vi "tui_LuaVIEW Task Manager.vi"() -> ()   [LabVIEW 2012]
doc: "This manager allows new tasks to be launched and existing tasks to be controlled and monitored. In case of a networked client/server setup, the tasks being managed are located on the server to which the client is connected."
uses:
  served/LuaVIEW Run or Swap Task_srv.ctl
  served/obj_LuaVIEW Task List_srv.ctl
  served/LuaVIEW Retrieve Scripts_srv.ctl
  served/LuaVIEW Info_srv.ctl
  served/re_LuaVIEW Kill Task_srv.ctl
  typedefs/t_LuaVIEW Task Manager Async Actions.ctl
  typedefs/t_LuaVIEW Task Manager States.ctl
  library/typedefs/t_Library Session Methods.ctl
  typedefs/clusters/LuaVIEW Task Console Ancillary.ctl
  typedefs/t_LuaVIEW Served Task List Methods.ctl
  typedefs/t_LuaVIEW Task Signals.ctl
  typedefs/t_LuaVIEW Task Modes.ctl
  clientsrv/typedefs/t_ClientSrv Access Levels.ctl
  library/glb_Library Configuration Globals.vi
panel:
  out "remote path cache":path
  out "remote file dialog":refnum<vi>
  in  "console":bool
  in  "swap remote":bool
  in  "swap local":bool
  in  "swap quick":bool
  out "kill task":T1
  in  "identifier":string
  out "info":T2
  out "retrieve scripts":T3
  in  "info":bool
  in  "run quick":bool
  in  "tabs":T4(tab)
  out "history content":string
  in  "insert new":bool
  in  "delete script":bool
  in  "next script":bool
  in  "previous script":bool
  in  "quick script history":string[](array[string])
  in  "script select":i32(ring)
  out "script":i32[](listbox)
  out "identifier":string
  in  "retrieve":bool
  out "handler":string
  out "swap time":string
  out "launch mode":enum16{"asynchronous", "manual", "synchronous"}(ring)
  out "deferred initialisation":bool
  out "priority":T5(ring)
  out "prefsys":T6(ring)
  out "task script on server":bool
  out "scripts":i32
  out "error":string
  in  "run remote":bool
  out "task list":T7
  out "run or swap task":T8
  out "local path cache":path
  in  "confirm":bool
  in  "kill":bool
  in  "run local":bool
  in  "stop":bool
  in  "resume":bool
  in  "pause":bool
  in  "task list":i32(listbox)
  in  "exit":bool
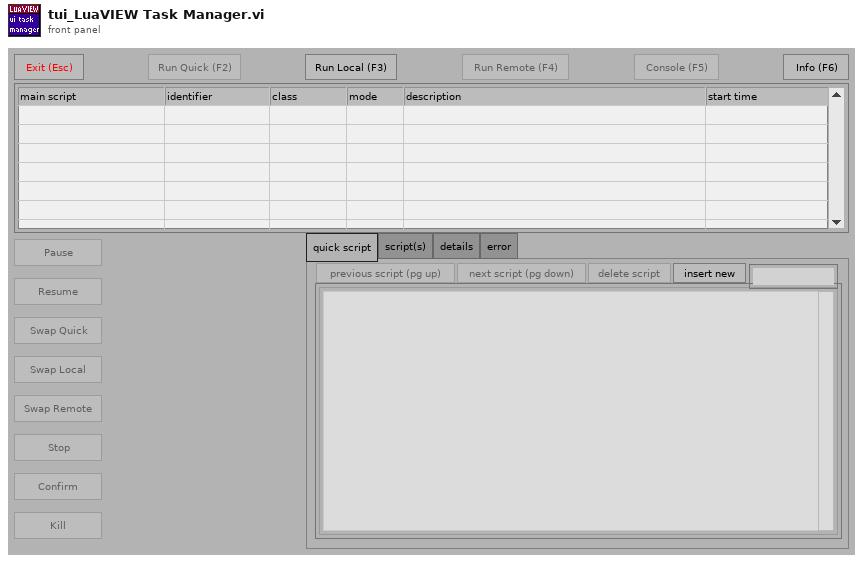
[diagram p1: front panel]
types:
  T1 = typedef "re_LuaVIEW Kill Task_srv.ctl" = refnum<vi>
  T2 = typedef "LuaVIEW Info_srv.ctl" = refnum<vi>
  T3 = typedef "LuaVIEW Retrieve Scripts_srv.ctl" = refnum<vi>
  T4 = enum32{"quick script", "script(s)", "details", "error"}
  T5 = enum32{"invalid priority", "background priority", "normal priority", "above normal priority", "high priority", "time critical priority", "subroutine"}
  T6 = enum32{"invalid execution system", "user interface", "standard", "instrument i/o", "data acquisition", "other 1", "other 2", "same as caller"}
  T7 = typedef "obj_LuaVIEW Task List_srv.ctl" = refnum<vi>
  T8 = typedef "LuaVIEW Run or Swap Task_srv.ctl" = refnum<vi>
  T9 = typedef "t_LuaVIEW Task Manager States.ctl" = enum16{"empty queue", "poll list", "reselect", "select", "resize", "pause task", "resume task", "stop task", "confirm error", "swap quick", "swap local", "swap remote", "kill task", "retrieve scripts", "select script", "quick ablement", "initialize", "init refs", "init remote dlg", "init persist", "init list", "init scripts", "cleanup", "stop"}
  T10 = typedef "t_LuaVIEW Task Manager Async Actions.ctl" = enum16{"run quick", "run local", "run remote", "stop"}
  T11 = typedef "t_ClientSrv Access Levels.ctl" = enum16{"observer", "operator", "local"}
  T12 = enum32{"existing file", "new file", "new or existing file", "existing dir", "new dir", "new or existing dir", "existing file (use LLBs)", "new file (use LLBs)", "new or existing file (use LLBs)", "new or existing file or directory (use LLBs)"}
  T13 = typedef "t_Library Session Methods.ctl" = enum16{"run", "get arg", "set arg", "delist", "cleanup?", "start session", "stop session", "list empty?"}
  T14 = typedef "LuaVIEW Task Console Ancillary.ctl" = cluster{"open on start":bool, "stop on close":bool, "hide initial":bool, "timeout":u32}
  T15 = typedef "t_LuaVIEW Served Task List Methods.ctl" = enum16{"get list", "resume", "pause", "swap", "stop", "confirm"}
  T16 = typedef "t_LuaVIEW Task Signals.ctl" = enum32{"resume", "pause", "swap", "stop", "confirm"}
  T17 = typedef "t_LuaVIEW Task Modes.ctl" = enum16{"initializing", "running", "executing", "paused", "error", "swapping"}
  T18 = typedef "eventvkey.ctl" = enum16{"ASCII", "Enter", "Return", "Shift", "Ctrl", "Alt", "Cmd", "Opt", "Caps", "NumLock", "Clear", "Break", "Up", "Down", "Left", "Right", "Insert", "Delete", "Home", "End", "PageUp", "PageDown", "Escape", "Help", "Pause", "ScrollLock", "F1", "F2", "F3", "F4", "F5", "F6", "F7", "F8", "F9", "F10", "F11", "F12", "F13", "F14", "F15", "F16", "F17", "F18", "F19", "F20", "F21", "F22", "F23", "F24", "Play", "VolumeUp", "VolumeDown", "Mute", "Two Byte Char"}
  T19 = typedef "LuaVIEW Task Info.ctl" = cluster{"main script":string, "identifier":string, "class":string, "description":string, "mode":T17, "handler":string, "LuaVIEW reference":T20, "scripts":i32, "hide":bool, "active":bool, "error msg":string, "defer":bool, "launch":enum16{"asynchronous", "manual", "synchronous"}, "main path valid":bool, "start time":dbl, "swap time":dbl, "task VI":refnum<vi>, "prefsys":enum32{"invalid execution system", "user interface", "standard", "instrument i/o", "data acquisition", "other 1", "other 2", "same as caller"}, "priority":enum32{"invalid priority", "background priority", "normal priority", "above normal priority", "high priority", "time critical priority", "subroutine"}, "signal flags":u32, "allow mask":u32, "handle mask":u32, "disallow manual":bool}
  T20 = typedef "t_LuaVIEW Reference.ctl" = refnum<k1>
  T21 = typedef "LuaVIEW Script Info.ctl" = cluster{"path":path, "description":string, "text":string, "parent index":i32, "version":string}
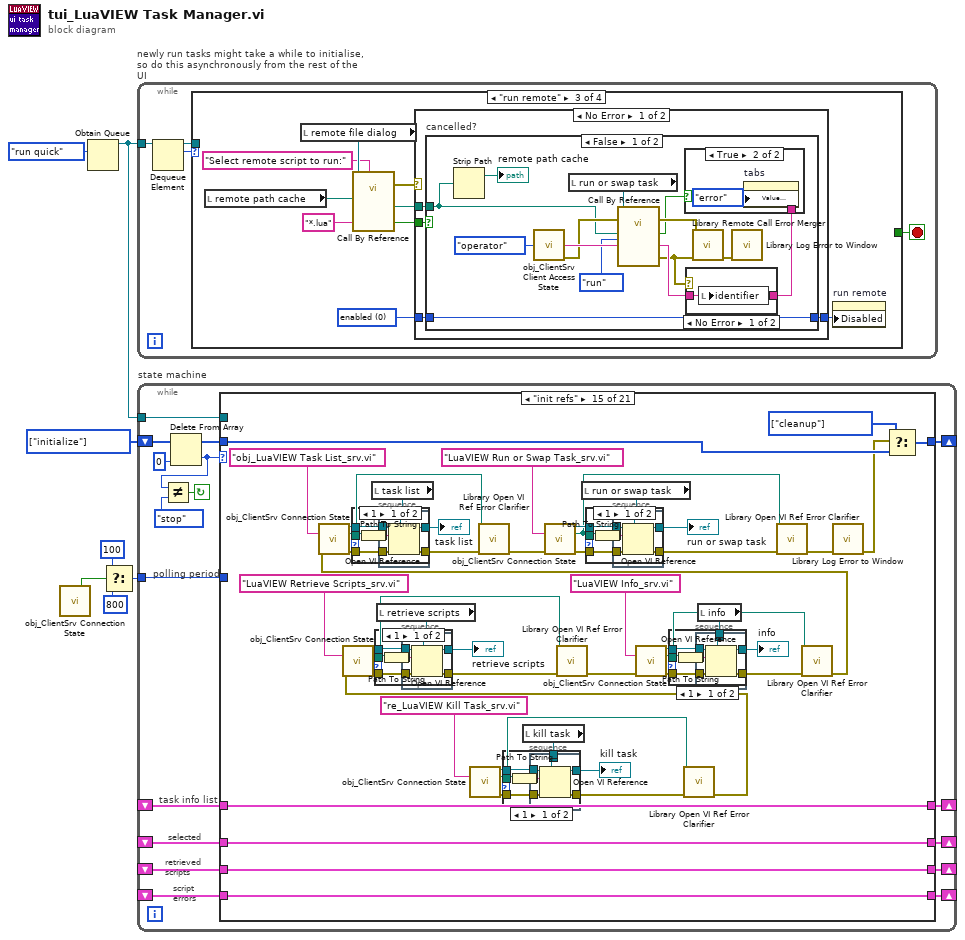
[diagram p0: block diagram]
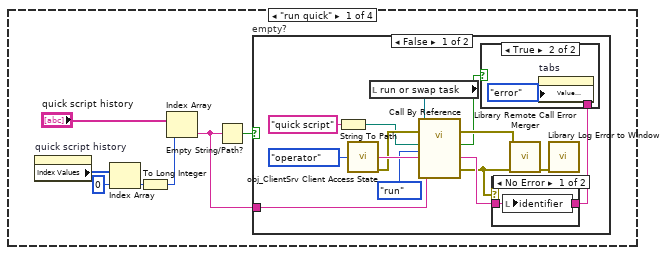
[diagram p2: hidden frame]
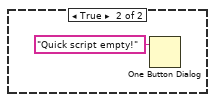
[diagram p5: hidden frame]
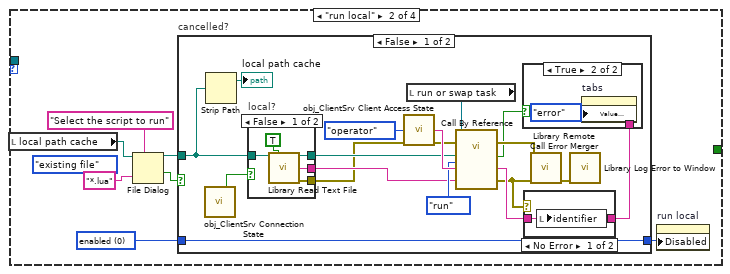
[diagram p6: hidden frame]
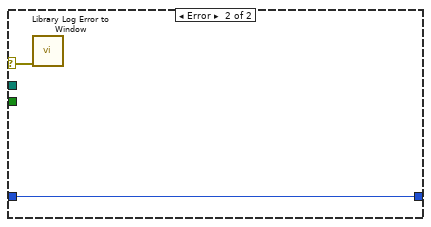
[diagram p14: hidden frame]
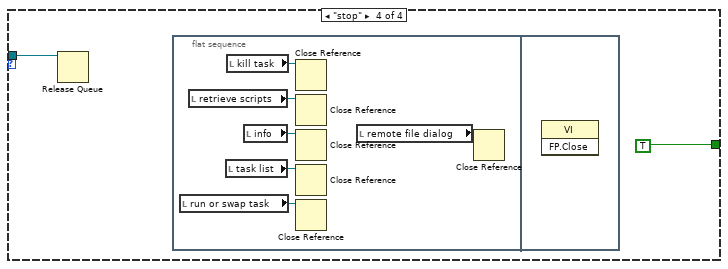
[diagram p15: hidden frame]
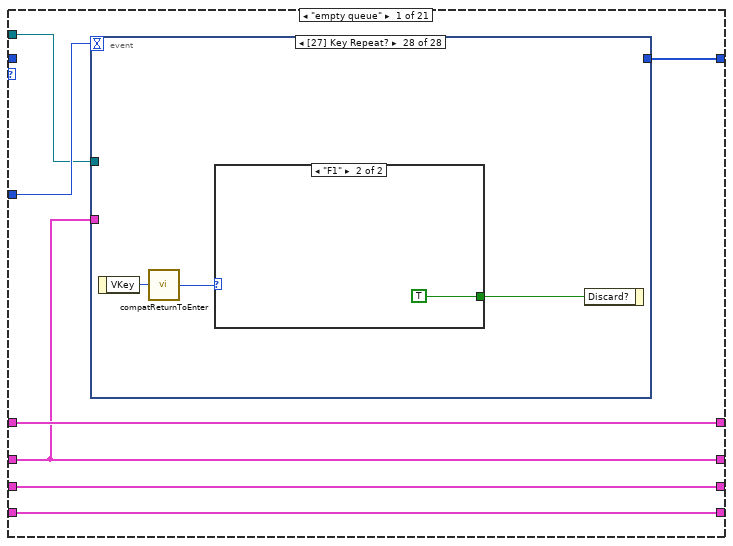
[diagram p16: hidden frame]
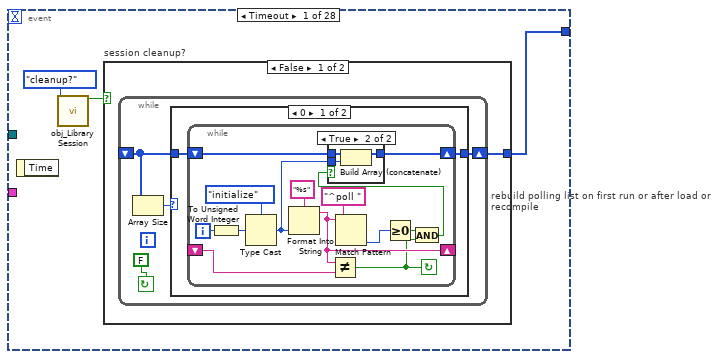
[diagram p17: hidden frame]
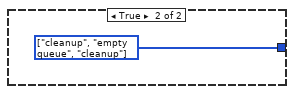
[diagram p20: hidden frame]
diagram:
  w7 = T9[] [enum."initialize"] items=["empty queue", "poll list", "reselect", "select", "resize", "pause task", "resume task", "stop task", "confirm error", "swap quick", "swap local", "swap remote", "kill task", "retrieve scripts", "select script", "quick ablement", "initialize", "init refs", "init remote dlg", "init persist", "init list", "init scripts", "cleanup", "stop"] ("Array Constant")
  n1 = call "obj_ClientSrv Connection State.vi"() -> ("local?"=w3:bool)  [unwired: 8 in, 7 out]
  n2 = Obtain Queue(element data type=t_LuaVIEW_Task_Manager_Async_Actions."run quick" ("actions")) -> (queue out=w6:refnum<queue>)  [unwired: 4 in, 2 out]
  n3 = Select(t=100, s=w3, f=800) -> (s? t:f=w2:i32)
  n4 = while "newly run tasks might take a while to initialise, so do this asynchronously from the rest of the UI" {
    tunnel: w6 -> [w11]
    stop <- w9 stop-if-true
    n5 = Dequeue Element(queue=w11) -> (queue out=w10:refnum<queue>, element=w8:T10)  [unwired: 2 in, 2 out]
    n6 = case "Case" shown="\"run remote\"" w8 {
      tunnel: w10 -> [_ _ _ w106]
      tunnel: [_ _ _ TRUE] -> w9
      frame "run quick" {
        n7 = property on="quick script history" class="Arr (strict)"() -> ("Index Values"=w18:u32[])  [unwired: 2 in, 2 out]
        n8 = Index Array(array=w18, index=0) -> (element=w15:u32)
        n9 = To Long Integer(number=w15) -> (32bit integer=w14:i32)
        n10 = Index Array(array="quick script history", index=w14) -> (element=w12:string)
        n11 = Empty String/Path?(string/path=w12) -> (empty?=w13:bool)
        n12 = case "empty?" shown="False" w13 {
          tunnel: w12 -> [w26 _]
          frame False {
            n13 = String To Path(string="quick script") -> (path=w24:path)
            n14 = call "obj_ClientSrv Client Access State.vi"("access level (observer)"=t_ClientSrv_Access_Levels."operator" ("access level in")) -> ("certificate"=w29:string, "error out"=w28:errorcluster)  [unwired: 13 in]
            n15 = local read "run or swap task"() -> (w27:T8)
            n16 = call-by-ref "?"(reference=w27, error in=w28, "script file or name (no name)"=w24, "action"=enum16{"run", "swap"}."run", "certificate"=w29, "script string (\"\" == load from file)"=w26) -> (error out=w32:errorcluster, "manual error"=w22:bool, "identifier"=w23:string, 15:"error out"=w21:errorcluster)  [unwired: 9 in, 1 out]
            n17 = case shown="No Error" w21 {
              tunnel: w23 -> [w33 w34]
              tunnel: [w33 w34] -> w20
              frame No Error {
                n18 = local write "identifier"(w33) -> ()
              }
              frame Error {
              }
            }
            n19 = case shown="True" w22 {
              tunnel: w20 -> [_ _]
              frame False {
              }
              frame True {
                n20 = property on="tabs" class="TabCtl (strict)"("Value (Signaling)"=T4."error") -> ()  [unwired: 2 in, 2 out]
              }
            }
            n21 = call "Library Remote Call Error Merger.vi"("call by reference node error"=w32, "called VI error (no error)"=w21) -> ("error out"=w31:errorcluster)  [unwired: 13 in]
            n22 = call "Library Log Error to Window.vi"("error in (no error)"=w31) -> ()  [unwired: 13 in, 2 out]
          }
          frame True {
            n23 = One Button Dialog(message="Quick script empty!") -> ()  [unwired: 1 in, 1 out]
          }
        }
      }
      frame "run local" {
        w37 = u8 0 items=["enabled", "disabled", "grayed"] ("disabled state")
        (unwired) T12."existing file" ("select mode (2)")
        n24 = local read "local path cache"() -> (w39:path)
        n25 = File Dialog(6:"*.lua" ("pattern"), 7:"Select the script to run" ("prompt (default)"), 11:w39) -> (1:w40:bool, 3:w41:path)  [unwired: 4 in, 2 out]
        n26 = case "cancelled?" shown="False" w40 {
          tunnel: w41 -> [w48 _]
          tunnel: w37 -> [w60 w71]
          tunnel: [w60 w71] -> w38
          frame False {
            n27 = call "obj_ClientSrv Connection State.vi"() -> ("local?"=w44:bool)  [unwired: 8 in, 7 out]
            n28 = Strip Path(path=w48) -> (stripped path=→"local path cache":path)  [unwired: 1 out]
            n29 = case "local?" shown="False" w44 {
              tunnel: w48 -> [w66 w67]
              tunnel: [w64 w67] -> w47
              tunnel: [w63 _] -> w46
              tunnel: [w62 _] -> w45
              frame False {
                n30 = call "Library Read Text File.vi"("file path"=w66, "convert eol (F)"=TRUE) -> ("dup path"=w64:path, "read text"=w63:string, "error out"=w62:errorcluster)  [unwired: 11 in]
              }
              frame True {
              }
            }
            n31 = call "obj_ClientSrv Client Access State.vi"("access level (observer)"=t_ClientSrv_Access_Levels."operator" ("access level in"), "error in (no error)"=w45) -> ("certificate"=w56:string, "error out"=w55:errorcluster)  [unwired: 12 in]
            n32 = local read "run or swap task"() -> (w54:T8)
            n33 = call-by-ref "?"(reference=w54, error in=w55, "script file or name (no name)"=w47, "action"=enum16{"run", "swap"}."run", "certificate"=w56, "script string (\"\" == load from file)"=w46) -> (error out=w59:errorcluster, "manual error"=w52:bool, "identifier"=w53:string, 15:"error out"=w50:errorcluster)  [unwired: 9 in, 1 out]
            n34 = case shown="No Error" w50 {
              tunnel: w53 -> [w68 w69]
              tunnel: [w68 w69] -> w51
              frame No Error {
                n35 = local write "identifier"(w68) -> ()
              }
              frame Error {
              }
            }
            n36 = case shown="True" w52 {
              tunnel: w51 -> [_ _]
              frame False {
              }
              frame True {
                n37 = property on="tabs" class="TabCtl (strict)"("Value (Signaling)"=T4."error") -> ()  [unwired: 2 in, 2 out]
              }
            }
            n38 = call "Library Remote Call Error Merger.vi"("call by reference node error"=w59, "called VI error (no error)"=w50) -> ("error out"=w58:errorcluster)  [unwired: 13 in]
            n39 = call "Library Log Error to Window.vi"("error in (no error)"=w58) -> ()  [unwired: 13 in, 2 out]
          }
          frame True {
          }
        }
        n40 = property on="run local" class="Bool"("Disabled"=w38) -> ()  [unwired: 2 in, 2 out]
      }
      frame "run remote" {
        w79 = u8 0 items=["enabled", "disabled", "grayed"] ("disabled state")
        n41 = local read "remote path cache"() -> (w75:path)
        n42 = local read "remote file dialog"() -> (w78:refnum<vi>)
        n43 = call-by-ref "?"(reference=w78, "prompt"="Select remote script to run:" ("prompt (default)"), "pattern"="*.lua", "start path"=w75) -> (error out=w77:errorcluster, "cancelled"=w74:bool, "path"=w72:path)  [unwired: 8 in, 1 out]
        n44 = case shown="No Error" w77 {
          selector: w77 -> [_ w103]
          tunnel: [w84 w104] -> w80
          tunnel: w79 -> [w83 w104]
          tunnel: w74 -> [w82 _]
          tunnel: w72 -> [w81 _]
          frame No Error {
            n45 = case "cancelled?" shown="False" w82 {
              tunnel: w83 -> [w97 w102]
              tunnel: [w97 w102] -> w84
              tunnel: w81 -> [w85 _]
              frame False {
                n46 = Strip Path(path=w85) -> (stripped path=→"remote path cache":path)  [unwired: 1 out]
                n47 = call "obj_ClientSrv Client Access State.vi"("access level (observer)"=t_ClientSrv_Access_Levels."operator" ("access level in")) -> ("certificate"=w93:string, "error out"=w92:errorcluster)  [unwired: 13 in]
                n48 = local read "run or swap task"() -> (w91:T8)
                n49 = call-by-ref "?"(reference=w91, error in=w92, "script file or name (no name)"=w85, "action"=enum16{"run", "swap"}."run", "certificate"=w93) -> (error out=w96:errorcluster, "manual error"=w89:bool, "identifier"=w90:string, 15:"error out"=w87:errorcluster)  [unwired: 10 in, 1 out]
                n50 = case shown="No Error" w87 {
                  tunnel: w90 -> [w99 w100]
                  tunnel: [w99 w100] -> w88
                  frame No Error {
                    n51 = local write "identifier"(w99) -> ()
                  }
                  frame Error {
                  }
                }
                n52 = case shown="True" w89 {
                  tunnel: w88 -> [_ _]
                  frame False {
                  }
                  frame True {
                    n53 = property on="tabs" class="TabCtl (strict)"("Value (Signaling)"=T4."error") -> ()  [unwired: 2 in, 2 out]
                  }
                }
                n54 = call "Library Remote Call Error Merger.vi"("call by reference node error"=w96, "called VI error (no error)"=w87) -> ("error out"=w95:errorcluster)  [unwired: 13 in]
                n55 = call "Library Log Error to Window.vi"("error in (no error)"=w95) -> ()  [unwired: 13 in, 2 out]
              }
              frame True {
              }
            }
          }
          frame Error {
            n56 = call "Library Log Error to Window.vi"("error in (no error)"=w103) -> ()  [unwired: 13 in, 2 out]
          }
        }
        n57 = property on="run remote" class="Bool"("Disabled"=w80) -> ()  [unwired: 2 in, 2 out]
      }
      frame "stop" {
        n58 = Release Queue(queue=w106) -> ()  [unwired: 2 in, 3 out]
        n59 = flat-sequence {
          frame #0 {
            n60 = local read "run or swap task"() -> (w111:T8)
            n61 = local read "retrieve scripts"() -> (w110:T3)
            n62 = local read "task list"() -> (w112:T7)
            n63 = local read "kill task"() -> (w108:T1)
            n64 = local read "info"() -> (w109:T2)
            n65 = Close Reference(reference=w108) -> ()  [unwired: 1 in, 1 out]
            n66 = Close Reference(reference=w110) -> ()  [unwired: 1 in, 1 out]
            n67 = Close Reference(reference=w109) -> ()  [unwired: 1 in, 1 out]
            n68 = Close Reference(reference=w112) -> ()  [unwired: 1 in, 1 out]
            n69 = Close Reference(reference=w111) -> ()  [unwired: 1 in, 1 out]
            n70 = local read "remote file dialog"() -> (w107:refnum<vi>)
            n71 = Close Reference(reference=w107) -> ()  [unwired: 1 in, 1 out]
          }
          frame #1 {
            n72 = invoke class="VI" method="FP.Close"() -> ()  [unwired: 3 in, 3 out]
          }
        }
      }
    }
  }
  n73 = while "state machine" {
    shift-left: w7 -> [w126]
    shift-right: [w129] -> _
    shift-right: [w122] -> _
    shift-left: _ -> [w123]
    shift-right: [w120] -> _
    shift-left: _ -> [w121]
    tunnel: w6 -> [w119]
    tunnel: w2 -> [w118]
    shift-right: [w116] -> _
    shift-left: _ -> [w117]
    shift-right: [w115] -> _
    shift-left: _ -> [w114]
    stop <- w128 continue-if-true
    # "script\nerrors"
    # "retrieved\nscripts"
    # "polling period"
    # "selected"
    # "task info list"
    n74 = Delete From Array(array=w126, index=0) -> (deleted portion=w113:T9, array with subset deleted=w125:T9[])  [unwired: 1 in]
    n75 = Not Equal?(x=w113, y=t_LuaVIEW_Task_Manager_States."stop" ("states")) -> (x != y?=w128:bool)
    n76 = case "Case" shown="\"init refs\"" w113 {
      selector: w113 -> [_ _ _ _ _ w563 _ _ _ _ _ _ _ _ _ _ _ _ _ _ _]
      tunnel: [w136 w351 w424 w438 w558 w574 w590 w622 w656 w676 w696 w734 w759 w780 w855 w962 w981 w989 w1002 w1018 w1027] -> w129
      tunnel: w125 -> [_ w352 w425 w438 w558 w574 w590 w622 w656 w677 w708 w734 w759 _ w853 w962 w982 w990 w1003 _ w1027]
      tunnel: w123 -> [w135 w358 w420 w437 w560 w575 w589 w621 w655 w678 w709 w733 w761 w782 w852 w968 w985 w992 w1005 w1012 w1026]
      tunnel: [w135 w359 w420 w437 w560 w575 w589 w621 w655 w678 w709 w733 w761 w782 w852 w968 w985 w992 w1005 w1012 w1020] -> w122
      tunnel: w121 -> [w130 w357 w426 _ w559 w561 w586 w613 w652 w675 w694 w732 w760 w781 w851 w967 w984 w991 w1004 w1017 w1025]
      tunnel: [w130 w357 w426 w435 w559 w561 w586 w613 w652 w675 w694 w732 w760 w781 w851 w967 w984 w991 w1004 w1017 w1025] -> w120
      tunnel: w119 -> [w131 _ _ _ _ _ _ _ _ _ _ _ _ _ _ _ _ _ _ _ w1024]
      tunnel: w118 -> [w134 _ _ _ _ _ _ _ _ _ _ _ _ _ _ _ _ _ _ _ _]
      tunnel: w117 -> [w133 w346 w422 w434 w556 w566 w588 w620 w654 w680 _ w731 w741 w779 w847 w966 w979 w987 w1000 w1014 w1023]
      tunnel: [w133 w346 w422 w434 w556 w566 w588 w620 w654 w680 w700 w731 w741 w779 w847 w966 w979 w987 w996 w1014 w1023] -> w116
      tunnel: [w132 w345 w421 w433 w555 w565 w587 w619 w653 w679 w699 w729 w740 w778 w845 w965 w978 w986 w994 w1013 w1022] -> w115
      tunnel: w114 -> [w132 w345 w421 w433 w555 w565 w587 w619 w653 w679 _ w729 w740 w778 w845 w965 w978 w986 w999 w1013 w1022]
      frame "empty queue" {
        n77 = event shown="[27] Key Repeat?" {
          selector: _ -> [_ _ _ _ _ _ _ _ _ _ _ _ _ _ _ _ _ _ _ _ _ _ _ _ _ _ _ _]
          dyn-events: _ -> [_ _ _ _ _ _ _ _ _ _ _ _ _ _ _ _ _ _ _ _ _ _ _ _ _ _ _ _]
          timeout: w134 -> [_ _ _ _ _ _ _ _ _ _ _ _ _ _ _ _ _ _ _ _ _ _ _ _ _ _ _ _]
          tunnel: [w139 w168 w170 _ w176 w179 w183 _ _ _ _ w222 w229 w236 w243 w251 w253 w266 w276 w292 w312 w314 w322 w323 w324 w325 w328 _] -> w136
          tunnel: w131 -> [_ _ _ w172 _ _ _ w185 w194 _ _ _ _ _ _ _ _ _ _ _ _ _ _ _ _ _ _ _]
          tunnel: w130 -> [_ _ _ _ _ _ _ _ _ w201 _ _ _ _ _ _ _ _ _ _ _ _ _ _ _ _ _ _]
          event Timeout {
            n78 = event-data() -> ()  [unwired: 1 in, 1 out]
            n79 = call "obj_Library Session.vi"("method"=t_Library_Session_Methods."cleanup?") -> ("cleanup/empty?"=w138:bool)  [unwired: 11 in, 3 out]
            n80 = case "session cleanup?" shown="False" w138 {
              tunnel: [w140 w166] -> w139
              frame False {
                n81 = while "rebuild polling list on first run or after load or recompile" {
                  shift-left: _ -> [w143]
                  shift-right: [w142] -> w140
                  stop <- FALSE continue-if-true
                  n82 = Array Size(array=w143) -> (size(s)=w144:i32)
                  n83 = case shown="0" w144 {
                    tunnel: [w145 w165] -> w142
                    tunnel: w143 -> [w146 w165]
                    frame 0 {
                      n84 = while {
                        shift-left: w146 -> [w155]
                        shift-right: [w153] -> w145
                        shift-left: _ -> [w157]
                        shift-right: [w152] -> _
                        i -> [w160]
                        stop <- w148 continue-if-true
                        n85 = To Unsigned Word Integer(number=w160) -> (unsigned 16bit integer=w158:u16)
                        n86 = Type Cast(type=t_LuaVIEW_Task_Manager_States."initialize" ("states"), x=w158) -> (*(type *) &x=w154:T9)
                        n87 = Format Into String(format string="%s" ("Format String"), w154) -> (resulting string=w152:string)  [unwired: 2 in, 1 out]
                        n88 = Not Equal?(x=w152, y=w157) -> (x != y?=w148:bool)
                        n89 = Match Pattern(string=w152, regular expression="^poll ") -> (offset past match=w150:i32)  [unwired: 1 in, 3 out]
                        n90 = Greater Or Equal To 0?(x=w150) -> (x >= 0?=w149:bool)
                        n91 = And(x=w149, y=w148) -> (x .and. y?=w147:bool)
                        n92 = case shown="True" w147 {
                          tunnel: w155 -> [w161 w164]
                          tunnel: w154 -> [_ w163]
                          tunnel: [w161 w162] -> w153
                          frame False {
                          }
                          frame True {
                            n93 = Build Array (concatenate)(w164, w163) -> (w162:T9[])
                          }
                        }
                      }
                    }
                    frame Default {
                    }
                  }
                }
              }
              frame True {
                w166 = T9[] [enum."cleanup", enum."empty queue", enum."cleanup"] items=["empty queue", "poll list", "reselect", "select", "resize", "pause task", "resume task", "stop task", "confirm error", "swap quick", "swap local", "swap remote", "kill task", "retrieve scripts", "select script", "quick ablement", "initialize", "init refs", "init remote dlg", "init persist", "init list", "init scripts", "cleanup", "stop"] ("Array Constant")
              }
            }
          }
          event Panel Close? {
            w168 = T9[] [enum."cleanup"] items=["empty queue", "poll list", "reselect", "select", "resize", "pause task", "resume task", "stop task", "confirm error", "swap quick", "swap local", "swap remote", "kill task", "retrieve scripts", "select script", "quick ablement", "initialize", "init refs", "init remote dlg", "init persist", "init list", "init scripts", "cleanup", "stop"] ("Array Constant")
            n94 = event-data() -> ()  [unwired: 1 in, 3 out]
            n95 = event-data("Discard?"=TRUE) -> ()  [unwired: 1 in, 1 out]
          }
          event "exit": Value Change {
            n96 = event-data() -> ()  [unwired: 1 in, 1 out]
            n97 = case shown="True" "exit" {
              tunnel: [w171 _] -> w170
              frame True {
                w171 = T9[] [enum."cleanup", enum."empty queue", enum."cleanup"] items=["empty queue", "poll list", "reselect", "select", "resize", "pause task", "resume task", "stop task", "confirm error", "swap quick", "swap local", "swap remote", "kill task", "retrieve scripts", "select script", "quick ablement", "initialize", "init refs", "init remote dlg", "init persist", "init list", "init scripts", "cleanup", "stop"] ("Array Constant")
              }
              frame False {
              }
            }
          }
          event "run quick": Value Change {
            n98 = event-data() -> ()  [unwired: 1 in, 5 out]
            n99 = case shown="True" "run quick" {
              tunnel: w172 -> [w175 _]
              frame True {
                n100 = Enqueue Element(queue=w175, element=t_LuaVIEW_Task_Manager_Async_Actions."run quick" ("states")) -> ()  [unwired: 2 in, 3 out]
              }
              frame False {
              }
            }
          }
          event "swap quick": Value Change {
            n101 = event-data() -> ()  [unwired: 1 in, 1 out]
            n102 = case shown="True" "swap quick" {
              tunnel: [w178 _] -> w176
              frame True {
                w178 = T9[] [enum."swap quick"] items=["empty queue", "poll list", "reselect", "select", "resize", "pause task", "resume task", "stop task", "confirm error", "swap quick", "swap local", "swap remote", "kill task", "retrieve scripts", "select script", "quick ablement", "initialize", "init refs", "init remote dlg", "init persist", "init list", "init scripts", "cleanup", "stop"] ("Array Constant")
              }
              frame False {
              }
            }
          }
          event "swap local": Value Change {
            n103 = event-data() -> ()  [unwired: 1 in, 1 out]
            n104 = case shown="True" "swap local" {
              tunnel: [w181 _] -> w179
              frame True {
                w181 = T9[] [enum."swap local"] items=["empty queue", "poll list", "reselect", "select", "resize", "pause task", "resume task", "stop task", "confirm error", "swap quick", "swap local", "swap remote", "kill task", "retrieve scripts", "select script", "quick ablement", "initialize", "init refs", "init remote dlg", "init persist", "init list", "init scripts", "cleanup", "stop"] ("Array Constant")
              }
              frame False {
              }
            }
          }
          event "swap remote": Value Change {
            n105 = event-data() -> ()  [unwired: 1 in, 1 out]
            n106 = case shown="True" "swap remote" {
              tunnel: [w184 _] -> w183
              frame True {
                w184 = T9[] [enum."swap remote"] items=["empty queue", "poll list", "reselect", "select", "resize", "pause task", "resume task", "stop task", "confirm error", "swap quick", "swap local", "swap remote", "kill task", "retrieve scripts", "select script", "quick ablement", "initialize", "init refs", "init remote dlg", "init persist", "init list", "init scripts", "cleanup", "stop"] ("Array Constant")
              }
              frame False {
              }
            }
          }
          event "run local": Value Change {
            n107 = event-data() -> ()  [unwired: 1 in, 5 out]
            n108 = case shown="True" "run local" {
              tunnel: w185 -> [w188 _]
              frame True {
                n109 = flat-sequence {
                  tunnel: w188 -> [w190]
                  tunnel: [w190] -> w187
                  tunnel: w187 -> [w192]
                  frame #0 {
                    w189 = u8 2 items=["enabled", "disabled", "grayed"] ("disabled state")
                    n110 = property on="run local" class="Bool"("Disabled"=w189) -> ()  [unwired: 2 in, 2 out]
                  }
                  frame #1 {
                    n111 = Enqueue Element(queue=w192, element=t_LuaVIEW_Task_Manager_Async_Actions."run local" ("states")) -> ()  [unwired: 2 in, 3 out]
                  }
                }
              }
              frame False {
              }
            }
          }
          event "run remote": Value Change {
            n112 = event-data() -> ()  [unwired: 1 in, 1 out]
            n113 = case shown="True" "run remote" {
              tunnel: w194 -> [w196 _]
              frame True {
                n114 = flat-sequence {
                  tunnel: w196 -> [w198]
                  tunnel: [w198] -> w195
                  tunnel: w195 -> [w200]
                  frame #0 {
                    w197 = u8 2 items=["enabled", "disabled", "grayed"] ("disabled state")
                    n115 = property on="run remote" class="Bool"("Disabled"=w197) -> ()  [unwired: 2 in, 2 out]
                  }
                  frame #1 {
                    n116 = Enqueue Element(queue=w200, element=t_LuaVIEW_Task_Manager_Async_Actions."run remote" ("states")) -> ()  [unwired: 2 in, 3 out]
                  }
                }
              }
              frame False {
              }
            }
          }
          event "console": Value Change {
            n117 = event-data() -> ()  [unwired: 1 in, 5 out]
            n118 = case shown="True" "console" {
              tunnel: w201 -> [w206 _]
              frame True {
                n119 = Unbundle By Name(w206) -> ("identifier"=w205:string)
                n120 = call "Library Resolve VI Path.vi"("VI name"="ui_LuaVIEW Task Console.vit", "sub path of toolkit (none)"=path "dynamic" ("subdirectory of tree (none)")) -> ("VI path"=w207:path)  [unwired: 13 in]
                n121 = Flatten To String(anything=T14 {"open on start"=TRUE, "stop on close"=TRUE, "hide initial"=FALSE, "timeout"=0} ("task console ancillary")) -> (data string=w203:string)  [unwired: 3 in, 2 out]
                n122 = call "obj_Library Session.vi"("method"=t_Library_Session_Methods."run", "path"=w207, "argument in (none)"=w205, "ancillary in (none)"=w203) -> ("error out"=w208:errorcluster)  [unwired: 8 in, 3 out]
                n123 = call "Library Log Error to Window.vi"("error in (no error)"=w208) -> ()  [unwired: 13 in, 2 out]
              }
              frame False {
              }
            }
          }
          event "info": Value Change {
            n124 = event-data() -> ()  [unwired: 1 in, 5 out]
            n125 = case shown="True" "info" {
              frame True {
                n126 = call "obj_ClientSrv Client Access State.vi"() -> ("certificate"=w218:string, "error out"=w217:errorcluster)  [unwired: 14 in]
                n127 = local read "info"() -> (w219:T2)
                n128 = call-by-ref "?"(reference=w219, error in=w217, "certificate"=w218) -> (error out=w215:errorcluster, "info"=w213:string, 15:"error out"=w216:errorcluster)  [unwired: 13 in, 1 out]
                n129 = call "Library Remote Call Error Merger.vi"("call by reference node error"=w215, "called VI error (no error)"=w216) -> ("error out"=w214:errorcluster)  [unwired: 13 in]
                n130 = case shown="No Error" w214 {
                  selector: w214 -> [_ w221]
                  tunnel: w213 -> [w220 _]
                  frame No Error {
                    n131 = One Button Dialog(message=w220) -> ()  [unwired: 1 in, 1 out]
                  }
                  frame Error {
                    n132 = call "Library Log Error to Window.vi"("error in (no error)"=w221) -> ()  [unwired: 13 in, 2 out]
                  }
                }
              }
              frame False {
              }
            }
          }
          event "pause": Value Change {
            n133 = event-data() -> ()  [unwired: 1 in, 5 out]
            n134 = case shown="True" "pause" {
              tunnel: [w227 _] -> w222
              frame True {
                w226 = u8 0 items=["enabled", "disabled", "grayed"] ("disabled state")
                n135 = property on="pause" class="Bool"() -> ("Disabled"=w225:u8)  [unwired: 2 in, 2 out]
                n136 = Equal?(x=w225, y=w226) -> (x = y?=w224:bool)
                n137 = case shown="True" w224 {
                  tunnel: [_ w228] -> w227
                  frame False {
                  }
                  frame True {
                    w228 = T9[] [enum."pause task"] items=["empty queue", "poll list", "reselect", "select", "resize", "pause task", "resume task", "stop task", "confirm error", "swap quick", "swap local", "swap remote", "kill task", "retrieve scripts", "select script", "quick ablement", "initialize", "init refs", "init remote dlg", "init persist", "init list", "init scripts", "cleanup", "stop"] ("Array Constant")
                  }
                }
              }
              frame False {
              }
            }
          }
          event "resume": Value Change {
            n138 = event-data() -> ()  [unwired: 1 in, 5 out]
            n139 = case shown="True" "resume" {
              tunnel: [w234 _] -> w229
              frame True {
                w233 = u8 0 items=["enabled", "disabled", "grayed"] ("disabled state")
                n140 = property on="resume" class="Bool"() -> ("Disabled"=w232:u8)  [unwired: 2 in, 2 out]
                n141 = Equal?(x=w232, y=w233) -> (x = y?=w231:bool)
                n142 = case shown="True" w231 {
                  tunnel: [_ w235] -> w234
                  frame False {
                  }
                  frame True {
                    w235 = T9[] [enum."resume task"] items=["empty queue", "poll list", "reselect", "select", "resize", "pause task", "resume task", "stop task", "confirm error", "swap quick", "swap local", "swap remote", "kill task", "retrieve scripts", "select script", "quick ablement", "initialize", "init refs", "init remote dlg", "init persist", "init list", "init scripts", "cleanup", "stop"] ("Array Constant")
                  }
                }
              }
              frame False {
              }
            }
          }
          event "stop": Value Change {
            n143 = event-data() -> ()  [unwired: 1 in, 5 out]
            n144 = case shown="True" "stop" {
              tunnel: [w241 _] -> w236
              frame True {
                w240 = u8 0 items=["enabled", "disabled", "grayed"] ("disabled state")
                n145 = property on="stop" class="Bool"() -> ("Disabled"=w239:u8)  [unwired: 2 in, 2 out]
                n146 = Equal?(x=w239, y=w240) -> (x = y?=w238:bool)
                n147 = case shown="True" w238 {
                  tunnel: [_ w242] -> w241
                  frame False {
                  }
                  frame True {
                    w242 = T9[] [enum."stop task"] items=["empty queue", "poll list", "reselect", "select", "resize", "pause task", "resume task", "stop task", "confirm error", "swap quick", "swap local", "swap remote", "kill task", "retrieve scripts", "select script", "quick ablement", "initialize", "init refs", "init remote dlg", "init persist", "init list", "init scripts", "cleanup", "stop"] ("Array Constant")
                  }
                }
              }
              frame False {
              }
            }
          }
          event "confirm": Value Change {
            n148 = event-data() -> ()  [unwired: 1 in, 5 out]
            n149 = case shown="True" "confirm" {
              tunnel: [w248 _] -> w243
              frame True {
                w247 = u8 0 items=["enabled", "disabled", "grayed"] ("disabled state")
                n150 = property on="confirm" class="Bool"() -> ("Disabled"=w246:u8)  [unwired: 2 in, 2 out]
                n151 = Equal?(x=w246, y=w247) -> (x = y?=w245:bool)
                n152 = case shown="True" w245 {
                  tunnel: [_ w249] -> w248
                  frame False {
                  }
                  frame True {
                    w249 = T9[] [enum."confirm error"] items=["empty queue", "poll list", "reselect", "select", "resize", "pause task", "resume task", "stop task", "confirm error", "swap quick", "swap local", "swap remote", "kill task", "retrieve scripts", "select script", "quick ablement", "initialize", "init refs", "init remote dlg", "init persist", "init list", "init scripts", "cleanup", "stop"] ("Array Constant")
                  }
                }
              }
              frame False {
              }
            }
          }
          event "kill": Value Change {
            n153 = event-data() -> ()  [unwired: 1 in, 5 out]
            n154 = case shown="True" "kill" {
              tunnel: [w252 _] -> w251
              frame True {
                w252 = T9[] [enum."kill task"] items=["empty queue", "poll list", "reselect", "select", "resize", "pause task", "resume task", "stop task", "confirm error", "swap quick", "swap local", "swap remote", "kill task", "retrieve scripts", "select script", "quick ablement", "initialize", "init refs", "init remote dlg", "init persist", "init list", "init scripts", "cleanup", "stop"] ("Array Constant")
              }
              frame False {
              }
            }
          }
          event "next script": Value Change {
            n155 = event-data() -> ()  [unwired: 1 in, 5 out]
            n156 = case shown="True" "next script" {
              tunnel: [w255 _] -> w253
              frame True {
                w255 = T9[] [enum."quick ablement"] items=["empty queue", "poll list", "reselect", "select", "resize", "pause task", "resume task", "stop task", "confirm error", "swap quick", "swap local", "swap remote", "kill task", "retrieve scripts", "select script", "quick ablement", "initialize", "init refs", "init remote dlg", "init persist", "init list", "init scripts", "cleanup", "stop"] ("Array Constant")
                n157 = local read "quick script history"() -> (w262:string[])
                n158 = property on="quick script history" class="Arr (strict)"() -> ("Index Values"=w264:u32[])  [unwired: 2 in, 2 out]
                n159 = Index Array(array=w264, index=0) -> (element=w263:u32)
                n160 = Array Size(array=w262) -> (size(s)=w261:i32)
                n161 = Increment(x=w263) -> (x+1=w258:u32)
                n162 = To Unsigned Long Integer(number=w261) -> (unsigned 32bit integer=w260:u32)
                n163 = Decrement(x=w260) -> (x-1=w259:u32)
                n164 = Max & Min(x=w259, y=w258) -> (min(x,y)=w257:u32)  [unwired: 1 out]
                n165 = Build Array(w257) -> (w256:u32[])
                n166 = property on="quick script history" class="Arr (strict)"("Index Values"=w256) -> ()  [unwired: 2 in, 2 out]
              }
              frame False {
              }
            }
          }
          event "previous script": Value Change {
            n167 = event-data() -> ()  [unwired: 1 in, 5 out]
            n168 = case shown="True" "previous script" {
              tunnel: [w268 _] -> w266
              frame True {
                w268 = T9[] [enum."quick ablement"] items=["empty queue", "poll list", "reselect", "select", "resize", "pause task", "resume task", "stop task", "confirm error", "swap quick", "swap local", "swap remote", "kill task", "retrieve scripts", "select script", "quick ablement", "initialize", "init refs", "init remote dlg", "init persist", "init list", "init scripts", "cleanup", "stop"] ("Array Constant")
                n169 = property on="quick script history" class="Arr (strict)"() -> ("Index Values"=w274:u32[])  [unwired: 2 in, 2 out]
                n170 = Index Array(array=w274, index=0) -> (element=w273:u32)
                n171 = Decrement(x=w273) -> (x-1=w272:u32)
                n172 = Max & Min(x=u32 0, y=w272) -> (max(x,y)=w269:u32)  [unwired: 1 out]
                n173 = Build Array(w269) -> (w271:u32[])
                n174 = property on="quick script history" class="Arr (strict)"("Index Values"=w271) -> ()  [unwired: 2 in, 2 out]
              }
              frame False {
              }
            }
          }
          event "delete script": Value Change {
            n175 = event-data() -> ()  [unwired: 1 in, 5 out]
            n176 = case shown="True" "delete script" {
              tunnel: [w287 _] -> w276
              frame True {
                w287 = T9[] [enum."quick ablement"] items=["empty queue", "poll list", "reselect", "select", "resize", "pause task", "resume task", "stop task", "confirm error", "swap quick", "swap local", "swap remote", "kill task", "retrieve scripts", "select script", "quick ablement", "initialize", "init refs", "init remote dlg", "init persist", "init list", "init scripts", "cleanup", "stop"] ("Array Constant")
                n177 = local read "quick script history"() -> (w288:string[])
                n178 = property on="quick script history" class="Arr (strict)"() -> ("Index Values"=w290:u32[])  [unwired: 2 in, 2 out]
                n179 = Index Array(array=w290, index=0) -> (element=w289:u32)
                n180 = To Long Integer(number=w289) -> (32bit integer=w284:i32)
                n181 = Delete From Array(array=w288, index=w284) -> (array with subset deleted=w286:string[])  [unwired: 1 in, 1 out]
                n182 = Array Size(array=w286) -> (size(s)=w285:i32)
                n183 = local write "quick script history"(w286) -> ()
                n184 = Decrement(x=w285) -> (x-1=w283:i32)
                n185 = Max & Min(x=w283, y=w284) -> (min(x,y)=w282:i32)  [unwired: 1 out]
                n186 = Max & Min(x=0, y=w282) -> (max(x,y)=w280:i32)  [unwired: 1 out]
                n187 = To Unsigned Long Integer(number=w280) -> (unsigned 32bit integer=w279:u32)
                n188 = Build Array(w279) -> (w278:u32[])
                n189 = property on="quick script history" class="Arr (strict)"("Index Values"=w278) -> ()  [unwired: 2 in, 2 out]
              }
              frame False {
              }
            }
          }
          event "insert new": Value Change {
            n190 = event-data() -> ()  [unwired: 1 in, 5 out]
            n191 = case shown="True" "insert new" {
              tunnel: [w296 _] -> w292
              frame True {
                w296 = T9[] [enum."quick ablement"] items=["empty queue", "poll list", "reselect", "select", "resize", "pause task", "resume task", "stop task", "confirm error", "swap quick", "swap local", "swap remote", "kill task", "retrieve scripts", "select script", "quick ablement", "initialize", "init refs", "init remote dlg", "init persist", "init list", "init scripts", "cleanup", "stop"] ("Array Constant")
                n192 = local read "quick script history"() -> (w299:string[])
                n193 = property on="quick script history" class="Arr (strict)"() -> ("Index Values"=w305:u32[])  [unwired: 2 in, 2 out]
                n194 = Index Array(array=w305, index=0) -> (element=w302:u32)
                n195 = Increment(x=w302) -> (x+1=w300:u32)
                n196 = Array Size(array=w299) -> (size(s)=w297:i32)
                n197 = To Long Integer(number=w300) -> (32bit integer=w298:i32)
                n198 = Max & Min(x=w297, y=w298) -> (min(x,y)=w295:i32)  [unwired: 1 out]
                n199 = To Unsigned Long Integer(number=w295) -> (unsigned 32bit integer=w294:u32)
                n200 = Insert Into Array(array=w299, index=w295, new element="" ("new element/subarray")) -> (w304:string[])
                n201 = Build Array(w294) -> (w301:u32[])
                n202 = stacked-sequence {
                  tunnel: w304 -> [w307 _ _]
                  tunnel: w301 -> [_ w308 _]
                  frame #0 {
                    n203 = local write "quick script history"(w307) -> ()
                  }
                  frame #1 {
                    n204 = property on="quick script history" class="Arr (strict)"("Index Values"=w308) -> ()  [unwired: 2 in, 2 out]
                  }
                  frame #2 {
                    n205 = property on="quick script history" class="Arr (strict)"() -> ("Array Element"=w310:refnum<vi>)  [unwired: 2 in, 2 out]
                    n206 = property class="Ctl"(reference=w310, "Key Focus"=TRUE) -> ()  [unwired: 1 in, 2 out]
                  }
                }
              }
              frame False {
              }
            }
          }
          event "retrieve": Value Change {
            n207 = event-data() -> ()  [unwired: 1 in, 1 out]
            n208 = case shown="True" "retrieve" {
              tunnel: [w313 _] -> w312
              frame True {
                w313 = T9[] [enum."retrieve scripts"] items=["empty queue", "poll list", "reselect", "select", "resize", "pause task", "resume task", "stop task", "confirm error", "swap quick", "swap local", "swap remote", "kill task", "retrieve scripts", "select script", "quick ablement", "initialize", "init refs", "init remote dlg", "init persist", "init list", "init scripts", "cleanup", "stop"] ("Array Constant")
              }
              frame False {
              }
            }
          }
          event "tabs": Value Change {
            n209 = event-data() -> ()  [unwired: 1 in, 6 out]
            n210 = case shown="\"error\"" "tabs" {
              tunnel: [_ w320 w321] -> w314
              frame Default {
                w316 = u8 2 items=["enabled", "disabled", "grayed"] ("disabled state")
                w317 = u8 2 items=["enabled", "disabled", "grayed"] ("disabled state")
                n211 = property on="run quick" class="Bool"("Disabled"=w317) -> ()  [unwired: 2 in, 2 out]
                n212 = property on="swap quick" class="Bool"("Disabled"=w316) -> ()  [unwired: 2 in, 2 out]
              }
              frame "error" {
                w318 = u8 2 items=["enabled", "disabled", "grayed"] ("disabled state")
                w320 = T9[] [enum."poll list"] items=["empty queue", "poll list", "reselect", "select", "resize", "pause task", "resume task", "stop task", "confirm error", "swap quick", "swap local", "swap remote", "kill task", "retrieve scripts", "select script", "quick ablement", "initialize", "init refs", "init remote dlg", "init persist", "init list", "init scripts", "cleanup", "stop"] ("Array Constant")
                w319 = u8 2 items=["enabled", "disabled", "grayed"] ("disabled state")
                n213 = property on="run quick" class="Bool"("Disabled"=w319) -> ()  [unwired: 2 in, 2 out]
                n214 = property on="swap quick" class="Bool"("Disabled"=w318) -> ()  [unwired: 2 in, 2 out]
              }
              frame "quick script" {
                w321 = T9[] [enum."quick ablement"] items=["empty queue", "poll list", "reselect", "select", "resize", "pause task", "resume task", "stop task", "confirm error", "swap quick", "swap local", "swap remote", "kill task", "retrieve scripts", "select script", "quick ablement", "initialize", "init refs", "init remote dlg", "init persist", "init list", "init scripts", "cleanup", "stop"] ("Array Constant")
              }
            }
          }
          event "quick script history": Value Change {
            w322 = T9[] [enum."quick ablement"] items=["empty queue", "poll list", "reselect", "select", "resize", "pause task", "resume task", "stop task", "confirm error", "swap quick", "swap local", "swap remote", "kill task", "retrieve scripts", "select script", "quick ablement", "initialize", "init refs", "init remote dlg", "init persist", "init list", "init scripts", "cleanup", "stop"] ("Array Constant")
            n215 = event-data() -> ()  [unwired: 1 in, 6 out]
          }
          event Panel Resize {
            w323 = T9[] [enum."resize"] items=["empty queue", "poll list", "reselect", "select", "resize", "pause task", "resume task", "stop task", "confirm error", "swap quick", "swap local", "swap remote", "kill task", "retrieve scripts", "select script", "quick ablement", "initialize", "init refs", "init remote dlg", "init persist", "init list", "init scripts", "cleanup", "stop"] ("Array Constant")
            n216 = event-data() -> ()  [unwired: 1 in, 8 out]
          }
          event "task list": Value Change {
            w324 = T9[] [enum."select"] items=["empty queue", "poll list", "reselect", "select", "resize", "pause task", "resume task", "stop task", "confirm error", "swap quick", "swap local", "swap remote", "kill task", "retrieve scripts", "select script", "quick ablement", "initialize", "init refs", "init remote dlg", "init persist", "init list", "init scripts", "cleanup", "stop"] ("Array Constant")
            n217 = event-data() -> ()  [unwired: 1 in, 6 out]
          }
          event "script select": Value Change {
            w325 = T9[] [enum."select script"] items=["empty queue", "poll list", "reselect", "select", "resize", "pause task", "resume task", "stop task", "confirm error", "swap quick", "swap local", "swap remote", "kill task", "retrieve scripts", "select script", "quick ablement", "initialize", "init refs", "init remote dlg", "init persist", "init list", "init scripts", "cleanup", "stop"] ("Array Constant")
            n218 = event-data() -> ()  [unwired: 1 in, 6 out]
          }
          event Key Down? {
            n219 = event-data() -> ("VKey"=w326:T18, "FocusObj"=w327:refnum<vi>)  [unwired: 1 in, 6 out]
            n220 = call <vilib>:"compatReturnToEnter.vi"("VKey"=w326) -> ("VKey"=w330:T18)
            n221 = case shown="\"Up\", \"Down\"" w330 {
              tunnel: [_ TRUE _] -> w329
              tunnel: [_ _ w337] -> w328
              tunnel: w327 -> [w332 _ _]
              frame "Up", "Down" {
                n222 = Type Cast(type=u32 0, x=w332) -> (*(type *) &x=w333:u32)
                n223 = Equal To 0?(x=w333) -> (x = 0?=w331:bool)
                n224 = case shown="True" w331 {
                  frame False {
                  }
                  frame True {
                    n225 = property on="task list" class="MCListbox (strict)"("Key Focus"=TRUE) -> ()  [unwired: 2 in, 2 out]
                  }
                }
              }
              frame "F1" {
                n226 = call "Library Show Help.vi"() -> ()  [unwired: 1 in]
              }
              frame Default {
                w337 = T9[] [enum."empty queue"] items=["empty queue", "poll list", "reselect", "select", "resize", "pause task", "resume task", "stop task", "confirm error", "swap quick", "swap local", "swap remote", "kill task", "retrieve scripts", "select script", "quick ablement", "initialize", "init refs", "init remote dlg", "init persist", "init list", "init scripts", "cleanup", "stop"] ("Array Constant")
              }
            }
            n227 = event-data("Discard?"=w329) -> ()  [unwired: 5 in, 1 out]
          }
          event event type 5.0.x8000000b {
            n228 = event-data() -> ("VKey"=w338:T18)  [unwired: 1 in]
            n229 = call <vilib>:"compatReturnToEnter.vi"("VKey"=w338) -> ("VKey"=w340:T18)
            n230 = case shown="\"F1\"" w340 {
              tunnel: [_ TRUE] -> w339
              frame Default {
              }
              frame "F1" {
              }
            }
            n231 = event-data("Discard?"=w339) -> ()  [unwired: 1 in, 1 out]
          }
        }
      }
      frame "poll list" {
        n232 = local read "task list"() -> (w349:T7)
        n233 = call "obj_ClientSrv Client Access State.vi"() -> ("certificate"=w344:string, "error out"=w353:errorcluster)  [unwired: 14 in]
        n234 = call-by-ref "?"(reference=w349, error in=w353, "method"=t_LuaVIEW_Served_Task_List_Methods."get list", "certificate"=w344) -> (error out=w354:errorcluster, "task info list"=w348:T19[], 15:"error out"=w343:errorcluster)  [unwired: 12 in, 1 out]
        n235 = Not Equal?(x=w348, y=w358) -> (x != y?=w355:bool)
        n236 = call "Library Remote Call Error Merger.vi"("call by reference node error"=w354, "called VI error (no error)"=w343) -> ("error out"=w347:errorcluster)  [unwired: 13 in]
        n237 = First Call?() -> (First Call?: T/F=w356:bool)
        n238 = Or(x=w355, y=w356) -> (x .or. y?=w350:bool)
        n239 = case shown="No Error" w347 {
          selector: w347 -> [_ w416]
          tunnel: [w365 w417] -> w359
          tunnel: w358 -> [w364 w417]
          tunnel: w348 -> [w363 _]
          tunnel: w352 -> [w361 _]
          tunnel: [w360 w418] -> w351
          tunnel: w350 -> [w362 _]
          frame No Error {
            n240 = case shown="True" w362 {
              tunnel: [w367 w372] -> w365
              tunnel: w363 -> [_ w372]
              tunnel: w364 -> [w367 w371]
              tunnel: w361 -> [w366 w369]
              tunnel: [w366 w370] -> w360
              frame False {
              }
              frame True {
                n241 = stacked-sequence {
                  tunnel: w372 -> [_ w376 w407 _]
                  tunnel: w371 -> [_ _ w406 _]
                  frame #0 {
                    n242 = property class="VI"() -> ("Front Panel"=w373:refnum<vi>)  [unwired: 2 in, 2 out]
                    n243 = property class="Pnl"(reference=w373, "Defer Panel Updates"=TRUE) -> ()  [unwired: 1 in, 2 out]
                  }
                  frame #1 {
                    n244 = for {
                      tunnel: w376 -> [w391] mode=indexing
                      tunnel: [w389] -> w375 mode=indexing
                      i -> [w385]
                      n245 = Unbundle By Name(w391) -> ("main script"=w378:string, "identifier"=w379:string, "class"=w380:string, "mode"=w382:T17, "description"=w388:string, "start time"=w387:dbl)
                      n246 = case shown="\"running\"" w382 {
                        tunnel: [u32 16744448 u32 15790320 u32 13828050 u32 13808820 u32 16727100 u32 16744448] -> w381
                        frame "initializing" {
                        }
                        frame "running" {
                        }
                        frame "executing" {
                        }
                        frame "paused" {
                        }
                        frame "error" {
                        }
                        frame "swapping" {
                        }
                      }
                      n247 = Bundle(w385, 3) -> (w383:cluster{i32, i32})  [unwired: 1 in]
                      n248 = global read "glb_Library Configuration Globals.vi" "time format"() -> (w377:string)
                      n249 = Format Date/Time String(time format string (%c)=w377, seconds (now)=w387) -> (date/time string=w386:string)  [unwired: 1 in]
                      n250 = Format Into String(w382) -> (resulting string=w390:string)  [unwired: 3 in, 1 out]
                      n251 = property on="task list" class="MCListbox (strict)"("Active Cell:Active Cell"=w383, "Active Cell:Cell Background Color"=w381) -> ()  [unwired: 2 in, 2 out]
                      n252 = Build Array(w378, w379, w380, w390, w388, w386) -> (w389:string[])
                    }
                    n253 = property on="task list" class="MCListbox (strict)"("Item Names"=w375) -> ()  [unwired: 2 in, 2 out]
                  }
                  frame #2 {
                    # "When tasks disappear from the list,\nmake sure the now empty cells\nare no longer coloured and the\nselection remains in range."
                    n254 = Array Size(array=w406) -> (size(s)=w405:i32)
                    n255 = Array Size(array=w407) -> (size(s)=w401:i32)
                    n256 = local read "task list"() -> (w403:i32)
                    n257 = Subtract(x=w405, y=w401) -> (x-y=w404:i32)
                    n258 = Decrement(x=w401) -> (x-1=w402:i32)
                    n259 = for {
                      N: w404 -> [_]
                      tunnel: w401 -> [w410]
                      i -> [w408]
                      n260 = Add(x=w410, y=w408) -> (x+y=w409:i32)
                      n261 = Bundle(w409, 3) -> (w412:cluster{i32, i32})  [unwired: 1 in]
                      n262 = property on="task list" class="MCListbox (strict)"("Active Cell:Active Cell"=w412, "Active Cell:Cell Background Color"=u32 15790320) -> ()  [unwired: 2 in, 2 out]
                    }
                    n263 = Max & Min(x=w402, y=w403) -> (min(x,y)=w400:i32)  [unwired: 1 out]
                    n264 = Max & Min(x=w400, y=0) -> (max(x,y)=w398:i32)  [unwired: 1 out]
                    n265 = local write "task list"(w398) -> ()
                  }
                  frame #3 {
                    n266 = property class="VI"() -> ("Front Panel"=w414:refnum<vi>)  [unwired: 2 in, 2 out]
                    n267 = property class="Pnl"(reference=w414, "Defer Panel Updates"=FALSE) -> ()  [unwired: 1 in, 2 out]
                  }
                }
                n268 = Build Array (concatenate)(t_LuaVIEW_Task_Manager_States."reselect" ("states"), w369) -> (w370:T9[])
              }
            }
          }
          frame Error {
            w418 = T9[] [enum."cleanup"] items=["empty queue", "poll list", "reselect", "select", "resize", "pause task", "resume task", "stop task", "confirm error", "swap quick", "swap local", "swap remote", "kill task", "retrieve scripts", "select script", "quick ablement", "initialize", "init refs", "init remote dlg", "init persist", "init list", "init scripts", "cleanup", "stop"] ("Array Constant")
            n269 = call "Library Log Error to Window.vi"("error in (no error)"=w416) -> ()  [unwired: 13 in, 2 out]
          }
        }
      }
      frame "reselect" {
        n270 = for {
          tunnel: w420 -> [w431] mode=indexing
          tunnel: "identifier" -> [w429]
          i -> [w427]
          n271 = Unbundle By Name(w431) -> ("identifier"=w430:string)
          n272 = Equal?(x=w429, y=w430) -> (x = y?=w428:bool)
          n273 = case shown="True" w428 {
            tunnel: w427 -> [_ w432]
            frame False {
            }
            frame True {
              n274 = local write "task list"(w432) -> ()
            }
          }
        }
        n275 = Build Array (concatenate)(t_LuaVIEW_Task_Manager_States."select" ("states"), w425) -> (w424:T9[])
      }
      frame "select" {
        n276 = Index Array(array=w437, index="task list") -> (element=w435:T19)
        n277 = stacked-sequence {
          tunnel: w435 -> [w439 w539 w551]
          frame #0 {
            n278 = while {
              tunnel: w439 -> [w452]
              shift-right: [w440] -> _
              shift-left: _ -> [w451]
              stop <- FALSE continue-if-true
              # "The confirm signal is exempted\nfrom being disallowed by the\n\"--#disallow_manual\" keyword."
              n279 = Unbundle By Name(w452) -> ("disallow manual"=w442:bool, "allow mask"=w446:u32)
              n280 = To Unsigned Long Integer(number=t_LuaVIEW_Task_Signals."confirm") -> (unsigned 32bit integer=w444:u32)
              n281 = Logical Shift(y=w444, x=u32 1) -> (x << y=w441:u32)
              n282 = case shown="True" w442 {
                tunnel: w446 -> [w453 w456]
                tunnel: w441 -> [_ w454]
                tunnel: [w453 w455] -> w440
                frame False {
                }
                frame True {
                  n283 = And(x=w454, y=w456) -> (x .and. y?=w455:u32)
                }
              }
              n284 = First Call?() -> (First Call?: T/F=w448:bool)
              n285 = Not Equal?(x=w440, y=w451) -> (x != y?=w449:bool)
              n286 = Or(x=w449, y=w448) -> (x .or. y?=w447:bool)
              n287 = case shown="True" w447 {
                tunnel: w440 -> [_ w457]
                frame False {
                }
                frame True {
                  n288 = stacked-sequence {
                    tunnel: w457 -> [w464 w474 w484 w494 w504 w514 w524]
                    frame #0 {
                      w460 = u8 0 items=["enabled", "disabled", "grayed"] ("disabled state")
                      w461 = u8 2 items=["enabled", "disabled", "grayed"] ("disabled state")
                      n289 = To Unsigned Long Integer(number=t_LuaVIEW_Task_Signals."pause") -> (unsigned 32bit integer=w466:u32)
                      n290 = Logical Shift(y=w466, x=u32 1) -> (x << y=w463:u32)
                      n291 = And(x=w463, y=w464) -> (x .and. y?=w462:u32)
                      n292 = Not Equal To 0?(x=w462) -> (x != 0?=w458:bool)
                      n293 = Select(t=w460, s=w458, f=w461) -> (s? t:f=w459:u8)
                      n294 = property on="pause" class="Bool"("Disabled"=w459) -> ()  [unwired: 2 in, 2 out]
                    }
                    frame #1 {
                      w470 = u8 0 items=["enabled", "disabled", "grayed"] ("disabled state")
                      w471 = u8 2 items=["enabled", "disabled", "grayed"] ("disabled state")
                      n295 = To Unsigned Long Integer(number=t_LuaVIEW_Task_Signals."resume") -> (unsigned 32bit integer=w476:u32)
                      n296 = Logical Shift(y=w476, x=u32 1) -> (x << y=w473:u32)
                      n297 = And(x=w473, y=w474) -> (x .and. y?=w472:u32)
                      n298 = Not Equal To 0?(x=w472) -> (x != 0?=w468:bool)
                      n299 = Select(t=w470, s=w468, f=w471) -> (s? t:f=w469:u8)
                      n300 = property on="resume" class="Bool"("Disabled"=w469) -> ()  [unwired: 2 in, 2 out]
                    }
                    frame #2 {
                      w481 = u8 2 items=["enabled", "disabled", "grayed"] ("disabled state")
                      n301 = To Unsigned Long Integer(number=t_LuaVIEW_Task_Signals."swap") -> (unsigned 32bit integer=w486:u32)
                      n302 = Logical Shift(y=w486, x=u32 1) -> (x << y=w483:u32)
                      n303 = property on="run quick" class="Bool"() -> ("Disabled"=w478:u8)  [unwired: 2 in, 2 out]
                      n304 = And(x=w483, y=w484) -> (x .and. y?=w482:u32)
                      n305 = Not Equal To 0?(x=w482) -> (x != 0?=w479:bool)
                      n306 = Select(t=w478, s=w479, f=w481) -> (s? t:f=w480:u8)
                      n307 = property on="swap quick" class="Bool"("Disabled"=w480) -> ()  [unwired: 2 in, 2 out]
                    }
                    frame #3 {
                      w490 = u8 0 items=["enabled", "disabled", "grayed"] ("disabled state")
                      w491 = u8 2 items=["enabled", "disabled", "grayed"] ("disabled state")
                      n308 = To Unsigned Long Integer(number=t_LuaVIEW_Task_Signals."swap") -> (unsigned 32bit integer=w496:u32)
                      n309 = Logical Shift(y=w496, x=u32 1) -> (x << y=w493:u32)
                      n310 = And(x=w493, y=w494) -> (x .and. y?=w492:u32)
                      n311 = Not Equal To 0?(x=w492) -> (x != 0?=w488:bool)
                      n312 = Select(t=w490, s=w488, f=w491) -> (s? t:f=w489:u8)
                      n313 = property on="swap local" class="Bool"("Disabled"=w489) -> ()  [unwired: 2 in, 2 out]
                    }
                    frame #4 {
                      w501 = u8 2 items=["enabled", "disabled", "grayed"] ("disabled state")
                      n314 = To Unsigned Long Integer(number=t_LuaVIEW_Task_Signals."swap") -> (unsigned 32bit integer=w506:u32)
                      n315 = Logical Shift(y=w506, x=u32 1) -> (x << y=w503:u32)
                      n316 = property on="run remote" class="Bool"() -> ("Disabled"=w498:u8)  [unwired: 2 in, 2 out]
                      n317 = And(x=w503, y=w504) -> (x .and. y?=w502:u32)
                      n318 = Not Equal To 0?(x=w502) -> (x != 0?=w499:bool)
                      n319 = Select(t=w498, s=w499, f=w501) -> (s? t:f=w500:u8)
                      n320 = property on="swap remote" class="Bool"("Disabled"=w500) -> ()  [unwired: 2 in, 2 out]
                    }
                    frame #5 {
                      w510 = u8 0 items=["enabled", "disabled", "grayed"] ("disabled state")
                      w511 = u8 2 items=["enabled", "disabled", "grayed"] ("disabled state")
                      n321 = To Unsigned Long Integer(number=t_LuaVIEW_Task_Signals."stop") -> (unsigned 32bit integer=w516:u32)
                      n322 = Logical Shift(y=w516, x=u32 1) -> (x << y=w513:u32)
                      n323 = And(x=w513, y=w514) -> (x .and. y?=w512:u32)
                      n324 = Not Equal To 0?(x=w512) -> (x != 0?=w508:bool)
                      n325 = Select(t=w510, s=w508, f=w511) -> (s? t:f=w509:u8)
                      n326 = property on="stop" class="Bool"("Disabled"=w509) -> ()  [unwired: 2 in, 2 out]
                    }
                    frame #6 {
                      w520 = u8 0 items=["enabled", "disabled", "grayed"] ("disabled state")
                      w521 = u8 2 items=["enabled", "disabled", "grayed"] ("disabled state")
                      n327 = To Unsigned Long Integer(number=t_LuaVIEW_Task_Signals."confirm") -> (unsigned 32bit integer=w526:u32)
                      n328 = Logical Shift(y=w526, x=u32 1) -> (x << y=w523:u32)
                      n329 = And(x=w523, y=w524) -> (x .and. y?=w522:u32)
                      n330 = Not Equal To 0?(x=w522) -> (x != 0?=w518:bool)
                      n331 = Select(t=w520, s=w518, f=w521) -> (s? t:f=w519:u8)
                      n332 = property on="confirm" class="Bool"("Disabled"=w519) -> ()  [unwired: 2 in, 2 out]
                    }
                  }
                }
              }
            }
          }
          frame #1 {
            w529 = u8 2 items=["enabled", "disabled", "grayed"] ("disabled state")
            w536 = u8 0 items=["enabled", "disabled", "grayed"] ("disabled state")
            n333 = Unbundle By Name(w539) -> ("mode"=w533:T17, "identifier"=w537:string, "hide"=w528:bool)
            n334 = Equal?(x=t_LuaVIEW_Task_Modes."error" ("mode"), y=w533) -> (x = y?=w534:bool)
            n335 = local write "identifier"(w537) -> ()
            n336 = Empty String/Path?(string/path=w537) -> (empty?=w538:bool)
            n337 = Select(t=w529, s=w538, f=w536) -> (s? t:f=w530:u8)
            n338 = Select(t=w529, s=w534, f=w530) -> (s? t:f=w535:u8)
            n339 = Select(t=w529, s=w528, f=w530) -> (s? t:f=w531:u8)
            n340 = property on="kill" class="Bool"("Disabled"=w535) -> ()  [unwired: 2 in, 2 out]
            n341 = property on="console" class="Bool"("Disabled"=w530) -> ()  [unwired: 2 in, 2 out]
            n342 = property on="retrieve" class="Bool"("Disabled"=w531) -> ()  [unwired: 2 in, 2 out]
          }
          frame #2 {
            n343 = Unbundle By Name(w551) -> ("error msg"=→"error":string, "scripts"=→"scripts":i32, "main path valid"=→"task script on server":bool, "prefsys"=→"prefsys":T6, "priority"=→"priority":T5, "defer"=→"deferred initialisation":bool, "launch"=→"launch mode":enum16{"asynchronous", "manual", "synchronous"}, "handler"=→"handler":string, "swap time"=w542:dbl)
            n344 = Not Equal To 0?(x=w542) -> (x != 0?=w543:bool)
            n345 = case shown="True" w543 {
              tunnel: w542 -> [_ w553]
              tunnel: [_ w552] -> w541
              frame False {
              }
              frame True {
                n346 = global read "glb_Library Configuration Globals.vi" "time format"() -> (w554:string)
                n347 = Format Date/Time String(time format string (%c)=w554, seconds (now)=w553) -> (date/time string=w552:string)  [unwired: 1 in]
              }
            }
            "swap time" <- w541
          }
        }
      }
      frame "resize" {
        n348 = control-ref of="task list"() -> (w557:refnum<vi>)
        n349 = call "Library MCListBox Resizer.vi"("MCListbox Refnum"=w557) -> ()  [unwired: 15 in]
      }
      frame "pause task".."confirm error" {
        n350 = case shown="\"confirm error\"" w563 {
          tunnel: [t_LuaVIEW_Served_Task_List_Methods."pause" ("method") t_LuaVIEW_Served_Task_List_Methods."resume" ("method") t_LuaVIEW_Served_Task_List_Methods."stop" ("method") t_LuaVIEW_Served_Task_List_Methods."confirm" ("method") t_LuaVIEW_Served_Task_List_Methods."get list" ("method")] -> w562
          frame "pause task" {
          }
          frame "resume task" {
          }
          frame "stop task" {
          }
          frame "confirm error" {
          }
          frame Default {
          }
        }
        n351 = call "obj_ClientSrv Client Access State.vi"("access level (observer)"=t_ClientSrv_Access_Levels."operator" ("access level in")) -> ("certificate"=w568:string, "error out"=w570:errorcluster)  [unwired: 13 in]
        n352 = Unbundle By Name(w561) -> ("identifier"=w567:string)
        n353 = local read "task list"() -> (w569:T7)
        n354 = call-by-ref "?"(reference=w569, error in=w570, "method"=w562, "certificate"=w568, "task identifier"=w567) -> (error out=w573:errorcluster, 15:"error out"=w564:errorcluster)  [unwired: 11 in, 2 out]
        n355 = call "Library Remote Call Error Merger.vi"("call by reference node error"=w573, "called VI error (no error)"=w564) -> ("error out"=w572:errorcluster)  [unwired: 13 in]
        n356 = call "Library Log Error to Window.vi"("error in (no error)"=w572) -> ()  [unwired: 13 in, 2 out]
      }
      frame "swap quick" {
        n357 = Unbundle By Name(w586) -> ("identifier"=w581:string)
        n358 = Format Into String(format string="Swap task \"%s\" with the visible quick script?" ("message"), w581) -> (resulting string=w584:string)  [unwired: 2 in, 1 out]
        n359 = Two Button Dialog(message=w584, 2:"Proceed" ("T button name (\"OK\")")) -> (T button?=w582:bool)  [unwired: 1 in]
        n360 = case shown="True" w582 {
          tunnel: w581 -> [_ w591]
          frame False {
          }
          frame True {
            n361 = local read "quick script history"() -> (w592:string[])
            n362 = property on="quick script history" class="Arr (strict)"() -> ("Index Values"=w593:u32[])  [unwired: 2 in, 2 out]
            n363 = Index Array(array=w593, index=0) -> (element=w595:u32)
            n364 = To Long Integer(number=w595) -> (32bit integer=w596:i32)
            n365 = Index Array(array=w592, index=w596) -> (element=w598:string)
            n366 = Empty String/Path?(string/path=w598) -> (empty?=w597:bool)
            n367 = case "empty?" shown="False" w597 {
              tunnel: w598 -> [w604 _]
              tunnel: w591 -> [w599 _]
              frame False {
                n368 = String To Path(string="quick script") -> (path=w602:path)
                n369 = call "obj_ClientSrv Client Access State.vi"("access level (observer)"=t_ClientSrv_Access_Levels."operator" ("access level in")) -> ("certificate"=w607:string, "error out"=w606:errorcluster)  [unwired: 13 in]
                n370 = local read "run or swap task"() -> (w605:T8)
                n371 = call-by-ref "?"(reference=w605, error in=w606, "script file or name (no name)"=w602, "action"=enum16{"run", "swap"}."swap", "certificate"=w607, "identifier (use keyword)"=w599, "script string (\"\" == load from file)"=w604) -> (error out=w610:errorcluster, 15:"error out"=w601:errorcluster)  [unwired: 8 in, 3 out]
                n372 = call "Library Remote Call Error Merger.vi"("call by reference node error"=w610, "called VI error (no error)"=w601) -> ("error out"=w609:errorcluster)  [unwired: 13 in]
                n373 = call "Library Log Error to Window.vi"("error in (no error)"=w609) -> ()  [unwired: 13 in, 2 out]
              }
              frame True {
                n374 = One Button Dialog(message="Quick script empty!") -> ()  [unwired: 1 in, 1 out]
              }
            }
          }
        }
      }
      frame "swap local" {
        (unwired) T12."existing file" ("select mode (2)")
        n375 = local read "local path cache"() -> (w618:path)
        n376 = Unbundle By Name(w613) -> ("identifier"=w612:string)
        n377 = File Dialog(6:"*.lua" ("pattern"), 7:"Select the script to swap with:" ("prompt (default)"), 11:w618) -> (1:w617:bool, 3:w616:path)  [unwired: 4 in, 2 out]
        n378 = case "cancelled?" shown="False" w617 {
          tunnel: w616 -> [w625 _]
          tunnel: w612 -> [w629 _]
          frame False {
            n379 = call "obj_ClientSrv Connection State.vi"() -> ("local?"=w627:bool)  [unwired: 8 in, 7 out]
            n380 = Strip Path(path=w625) -> (stripped path=w628:path)  [unwired: 1 out]
            n381 = case "local?" shown="False" w627 {
              tunnel: w625 -> [w642 w643]
              tunnel: [w640 w643] -> w626
              tunnel: [w639 _] -> w624
              tunnel: [w638 _] -> w623
              frame False {
                n382 = call "Library Read Text File.vi"("file path"=w642, "convert eol (F)"=TRUE) -> ("dup path"=w640:path, "read text"=w639:string, "error out"=w638:errorcluster)  [unwired: 11 in]
              }
              frame True {
              }
            }
            n383 = local write "local path cache"(w628) -> ()
            n384 = call "obj_ClientSrv Client Access State.vi"("access level (observer)"=t_ClientSrv_Access_Levels."operator" ("access level in"), "error in (no error)"=w623) -> ("certificate"=w634:string, "error out"=w633:errorcluster)  [unwired: 12 in]
            n385 = local read "run or swap task"() -> (w632:T8)
            n386 = call-by-ref "?"(reference=w632, error in=w633, "script file or name (no name)"=w626, "action"=enum16{"run", "swap"}."swap", "certificate"=w634, "identifier (use keyword)"=w629, "script string (\"\" == load from file)"=w624) -> (error out=w637:errorcluster, 15:"error out"=w631:errorcluster)  [unwired: 8 in, 3 out]
            n387 = call "Library Remote Call Error Merger.vi"("call by reference node error"=w637, "called VI error (no error)"=w631) -> ("error out"=w636:errorcluster)  [unwired: 13 in]
            n388 = call "Library Log Error to Window.vi"("error in (no error)"=w636) -> ()  [unwired: 13 in, 2 out]
          }
          frame True {
          }
        }
      }
      frame "swap remote" {
        n389 = local read "remote path cache"() -> (w649:path)
        n390 = local read "remote file dialog"() -> (w647:refnum<vi>)
        n391 = Unbundle By Name(w652) -> ("identifier"=w651:string)
        n392 = call-by-ref "?"(reference=w647, "prompt"="Select remote script to swap with:" ("prompt (default)"), "pattern"="*.lua", "start path"=w649) -> (error out=w646:errorcluster, "cancelled"=w644:bool, "path"=w645:path)  [unwired: 8 in, 1 out]
        n393 = case shown="No Error" w646 {
          selector: w646 -> [_ w671]
          tunnel: w651 -> [w659 _]
          tunnel: w645 -> [w658 _]
          tunnel: w644 -> [w657 _]
          frame No Error {
            n394 = case "cancelled?" shown="False" w657 {
              tunnel: w658 -> [w660 _]
              tunnel: w659 -> [w662 _]
              frame False {
                n395 = Strip Path(path=w660) -> (stripped path=w661:path)  [unwired: 1 out]
                n396 = local write "remote path cache"(w661) -> ()
                n397 = call "obj_ClientSrv Client Access State.vi"("access level (observer)"=t_ClientSrv_Access_Levels."operator" ("access level in")) -> ("certificate"=w667:string, "error out"=w666:errorcluster)  [unwired: 13 in]
                n398 = local read "run or swap task"() -> (w665:T8)
                n399 = call-by-ref "?"(reference=w665, error in=w666, "script file or name (no name)"=w660, "action"=enum16{"run", "swap"}."swap", "certificate"=w667, "identifier (use keyword)"=w662) -> (error out=w670:errorcluster, 15:"error out"=w664:errorcluster)  [unwired: 9 in, 3 out]
                n400 = call "Library Remote Call Error Merger.vi"("call by reference node error"=w670, "called VI error (no error)"=w664) -> ("error out"=w669:errorcluster)  [unwired: 13 in]
                n401 = call "Library Log Error to Window.vi"("error in (no error)"=w669) -> ()  [unwired: 13 in, 2 out]
              }
              frame True {
              }
            }
          }
          frame Error {
            n402 = call "Library Log Error to Window.vi"("error in (no error)"=w671) -> ()  [unwired: 13 in, 2 out]
          }
        }
      }
      frame "kill task" {
        n403 = Unbundle By Name(w675) -> ("identifier"=w672:string)
        n404 = Format Into String(format string="Are you sure that task \"%s\" must be killed?\nKilling a task might interrupt some critical operation\nand prevent the cleanup of resources. Before killing\na task, make sure that it cannot be stopped." ("message"), w672) -> (resulting string=w674:string)  [unwired: 2 in, 1 out]
        n405 = Two Button Dialog(message=w674, 2:"Proceed" ("T button name (\"OK\")")) -> (T button?=w682:bool)  [unwired: 1 in]
        n406 = case shown="True" w682 {
          tunnel: w677 -> [w683 _]
          tunnel: [w683 w685] -> w676
          tunnel: w672 -> [_ w684]
          frame False {
          }
          frame True {
            w685 = T9[] [enum."poll list"] items=["empty queue", "poll list", "reselect", "select", "resize", "pause task", "resume task", "stop task", "confirm error", "swap quick", "swap local", "swap remote", "kill task", "retrieve scripts", "select script", "quick ablement", "initialize", "init refs", "init remote dlg", "init persist", "init list", "init scripts", "cleanup", "stop"] ("Array Constant")
            n407 = flat-sequence {
              tunnel: w684 -> [w686]
              frame #0 {
                n408 = call <vilib>:"Set Busy.vi"() -> ()  [unwired: 10 in, 2 out]
              }
              frame #1 {
                n409 = call "obj_ClientSrv Client Access State.vi"("access level (observer)"=t_ClientSrv_Access_Levels."operator" ("access level in")) -> ("certificate"=w689:string, "error out"=w691:errorcluster)  [unwired: 13 in]
                n410 = local read "kill task"() -> (w690:T1)
                n411 = call-by-ref "?"(reference=w690, error in=w691, "certificate"=w689, "task identifier"=w686) -> (error out=w688:errorcluster, 15:"error out"=w687:errorcluster)  [unwired: 13 in, 1 out]
                n412 = call "Library Remote Call Error Merger.vi"("call by reference node error"=w688, "called VI error (no error)"=w687) -> ("error out"=w693:errorcluster)  [unwired: 13 in]
                n413 = call "Library Log Error to Window.vi"("error in (no error)"=w693) -> ()  [unwired: 13 in, 2 out]
              }
              frame #2 {
                n414 = call <vilib>:"Unset Busy.vi"() -> ()  [unwired: 11 in, 1 out]
              }
            }
          }
        }
      }
      frame "retrieve scripts" {
        n415 = Unbundle By Name(w694) -> ("identifier"=w701:string)
        "identifier" <- w701
        n416 = call "obj_ClientSrv Client Access State.vi"() -> ("certificate"=w703:string, "error out"=w705:errorcluster)  [unwired: 14 in]
        n417 = local read "retrieve scripts"() -> (w704:T3)
        n418 = call-by-ref "?"(reference=w704, error in=w705, "certificate"=w703, "identifier"=w701) -> (error out=w707:errorcluster, "script infos"=w700:T21[], "script errors"=w699:cluster{"line numbers":i32[]}[], 15:"error out"=w702:errorcluster)  [unwired: 11 in, 1 out]
        n419 = for {
          tunnel: w700 -> [w715] mode=indexing
          tunnel: [w713] -> w698 mode=indexing
          n420 = Unbundle By Name(w715) -> ("path"=w714:path)
          n421 = Strip Path(path=w714) -> (stripped path=w710:path, name=w711:string)
          n422 = Empty String/Path?(string/path=w710) -> (empty?=w712:bool)
          n423 = case shown="False" w712 {
            tunnel: [w718 w721] -> w713
            tunnel: w711 -> [w719 w721]
            tunnel: w710 -> [w720 _]
            frame False {
              n424 = Path To String(path=w720) -> (string=w716:string)
              n425 = Concatenate Strings(w719, " in " ("string"), w716) -> (w718:string)
            }
            frame True {
            }
          }
        }
        n426 = call "Library Remote Call Error Merger.vi"("call by reference node error"=w707, "called VI error (no error)"=w702) -> ("error out"=w706:errorcluster)  [unwired: 13 in]
        n427 = call "Library Log Error to Window.vi"("error in (no error)"=w706) -> ()  [unwired: 13 in, 2 out]
        n428 = property on="script select" class="Ring (strict)"("Strings []"=w698, "Value"=0) -> ()  [unwired: 2 in, 2 out]
        n429 = Build Array (concatenate)(t_LuaVIEW_Task_Manager_States."select script" ("states"), w708) -> (w696:T9[])
      }
      frame "select script" {
        n430 = Index Array(array=w731, index="script select") -> (element=w725:T21)
        n431 = Index Array(array=w729, index="script select") -> (element=w728:cluster{"line numbers":i32[]})
        n432 = Unbundle By Name(w728) -> ("line numbers"=w727:i32[])
        n433 = Unbundle By Name(w725) -> ("text"=w724:string)
        n434 = call "Library Extract String Lines.vi"("multi-line string"=w724) -> ("lines"=w723:string[])  [unwired: 14 in]
        n435 = Decrement(x=w727) -> (x-1=w726:i32[])
        n436 = flat-sequence {
          tunnel: w726 -> [w735]
          tunnel: w723 -> [w736]
          tunnel: [w735] -> w722
          tunnel: w722 -> [w737]
          frame #0 {
            n437 = property on="script" class="LstBox (strict)"("Item Names"=w736) -> ()  [unwired: 2 in, 2 out]
          }
          frame #1 {
            "script" <- w737
          }
        }
      }
      frame "quick ablement" {
        n438 = local read "quick script history"() -> (w758:string[])
        n439 = property on="quick script history" class="Arr (strict)"() -> ("Index Values"=w750:u32[])  [unwired: 2 in, 2 out]
        n440 = Index Array(array=w750, index=0) -> (element=w743:u32)
        n441 = Array Size(array=w758) -> (size(s)=w745:i32)
        n442 = Increment(x=w743) -> (x+1=w744:u32)
        n443 = To Unsigned Long Integer(number=w745) -> (unsigned 32bit integer=w742:u32)
        n444 = Decrement(x=w745) -> (x-1=w757:i32)
        n445 = local read "tabs"() -> (w755:T4)
        n446 = Equal To 0?(x=w745) -> (x = 0?=w739:bool)
        n447 = To Unsigned Long Integer(number=w757) -> (unsigned 32bit integer=w749:u32)
        n448 = Max & Min(x=w742, y=w744) -> (min(x,y)=w746:u32)  [unwired: 1 out]
        n449 = case shown="\"quick script\"" w755 {
          tunnel: [w771 w774] -> w756
          tunnel: w739 -> [_ w773]
          tunnel: [w771 w772] -> w738
          frame Default {
            w771 = u8 2 items=["enabled", "disabled", "grayed"] ("disabled state")
          }
          frame "quick script" {
            n450 = case shown="False" w773 {
              tunnel: [w775 w777] -> w774
              tunnel: [w775 w776] -> w772
              frame True {
                w775 = u8 2 items=["enabled", "disabled", "grayed"] ("disabled state")
              }
              frame False {
                w777 = u8 0 items=["enabled", "disabled", "grayed"] ("disabled state")
                n451 = property on="swap local" class="Bool"() -> ("Disabled"=w776:u8)  [unwired: 2 in, 2 out]
              }
            }
          }
        }
        n452 = Format Into String(format string="%d/%d", w746, w742) -> (resulting string=→"history content":string)  [unwired: 2 in, 1 out]
        n453 = property on="run quick" class="Bool"("Disabled"=w756) -> ()  [unwired: 2 in, 2 out]
        n454 = property on="swap quick" class="Bool"("Disabled"=w738) -> ()  [unwired: 2 in, 2 out]
        n455 = case "empty history" shown="False" w739 {
          tunnel: [w767 w770] -> w754
          tunnel: [w769 w770] -> w753
          tunnel: [w768 w770] -> w752
          tunnel: w743 -> [w763 _]
          tunnel: w749 -> [w764 _]
          frame False {
            w766 = u8 2 items=["enabled", "disabled", "grayed"] ("disabled state")
            w767 = u8 0 items=["enabled", "disabled", "grayed"] ("disabled state")
            n456 = Greater?(x=w764, y=w763) -> (0:w762:bool)
            n457 = Greater Than 0?(x=w763) -> (x > 0?=w765:bool)
            n458 = Select(t=w767, s=w762, f=w766) -> (s? t:f=w769:u8)
            n459 = Select(t=w767, s=w765, f=w766) -> (s? t:f=w768:u8)
          }
          frame True {
            w770 = u8 2 items=["enabled", "disabled", "grayed"] ("disabled state")
          }
        }
        n460 = property on="delete script" class="Bool"("Disabled"=w754) -> ()  [unwired: 2 in, 2 out]
        n461 = property on="next script" class="Bool"("Disabled"=w753) -> ()  [unwired: 2 in, 2 out]
        n462 = property on="previous script" class="Bool"("Disabled"=w752) -> ()  [unwired: 2 in, 2 out]
      }
      frame "initialize" {
        n463 = while "rebuild init list on first run or after load or recompile" {
          shift-left: _ -> [w785]
          shift-right: [w784] -> w780
          stop <- FALSE continue-if-true
          n464 = Array Size(array=w785) -> (size(s)=w786:i32)
          n465 = case shown="0" w786 {
            tunnel: [w787 w807] -> w784
            tunnel: w785 -> [w788 w807]
            frame 0 {
              n466 = while {
                shift-left: w788 -> [w797]
                shift-right: [w795] -> w787
                shift-left: _ -> [w799]
                shift-right: [w794] -> _
                i -> [w802]
                stop <- w790 continue-if-true
                n467 = To Unsigned Word Integer(number=w802) -> (unsigned 16bit integer=w800:u16)
                n468 = Type Cast(type=t_LuaVIEW_Task_Manager_States."initialize" ("states"), x=w800) -> (*(type *) &x=w796:T9)
                n469 = Format Into String(format string="%s" ("Format String"), w796) -> (resulting string=w794:string)  [unwired: 2 in, 1 out]
                n470 = Not Equal?(x=w794, y=w799) -> (x != y?=w790:bool)
                n471 = Match Pattern(string=w794, regular expression="^init ") -> (offset past match=w792:i32)  [unwired: 1 in, 3 out]
                n472 = Greater Or Equal To 0?(x=w792) -> (x >= 0?=w791:bool)
                n473 = And(x=w791, y=w790) -> (x .and. y?=w789:bool)
                n474 = case shown="True" w789 {
                  tunnel: w797 -> [w803 w806]
                  tunnel: w796 -> [_ w805]
                  tunnel: [w803 w804] -> w795
                  frame False {
                  }
                  frame True {
                    n475 = Build Array (concatenate)(w806, w805) -> (w804:T9[])
                  }
                }
              }
            }
            frame Default {
            }
          }
        }
      }
      frame "init refs" {
        w854 = T9[] [enum."cleanup"] items=["empty queue", "poll list", "reselect", "select", "resize", "pause task", "resume task", "stop task", "confirm error", "swap quick", "swap local", "swap remote", "kill task", "retrieve scripts", "select script", "quick ablement", "initialize", "init refs", "init remote dlg", "init persist", "init list", "init scripts", "cleanup", "stop"] ("Array Constant")
        n476 = local read "task list"() -> (w830:T7)
        n477 = local read "retrieve scripts"() -> (w814:T3)
        n478 = call "obj_ClientSrv Connection State.vi"("machine{connect}/VI{get state} name (local/no path resolution)"="re_LuaVIEW Kill Task_srv.vi") -> ("server app ref"=w810:refnum<vi>, "resolved server path"=w809:path, "error out"=w808:errorcluster)  [unwired: 7 in, 5 out]
        n479 = local read "kill task"() -> (w812:T1)
        n480 = stacked-sequence {
          tunnel: [w861] -> w811
          tunnel: [w860] -> w813
          tunnel: w808 -> [w859]
          tunnel: w810 -> [w858]
          tunnel: w809 -> [w857]
          tunnel: w812 -> [w856]
          frame #0 {
            # "avoid LV8 complaints"
            n481 = Path to Array of Strings(0:w857) -> (2:w862:string[])  [unwired: 1 out]
            n482 = Array Size(array=w862) -> (size(s)=w863:i32)
            n483 = case shown="1" w863 {
              tunnel: w857 -> [w870 w876]
              tunnel: w858 -> [w868 w875]
              tunnel: [w866 w871] -> w861
              tunnel: [w864 w874] -> w860
              tunnel: w856 -> [w865 w873]
              tunnel: w859 -> [w867 w872]
              frame 1 {
                n484 = Path To String(path=w870) -> (string=w869:string)
                n485 = Open VI Reference(type specifier VI Refnum (for type only)=w865, application reference (local)=w868, vi path=w869, error in (no error)=w867) -> (vi reference=w866:T1, error out=w864:errorcluster)  [unwired: 2 in]
              }
              frame Default {
                n486 = Open VI Reference(type specifier VI Refnum (for type only)=w873, application reference (local)=w875, vi path=w876, error in (no error)=w872) -> (vi reference=w871:T1, error out=w874:errorcluster)  [unwired: 2 in]
              }
            }
          }
        }
        "kill task" <- w811
        n487 = local read "run or swap task"() -> (w835:T8)
        n488 = call "Library Open VI Ref Error Clarifier.vi"("VI path"=w809, "called VI error (no error)"=w813) -> ("error out"=w838:errorcluster)  [unwired: 13 in]
        n489 = call "obj_ClientSrv Connection State.vi"("machine{connect}/VI{get state} name (local/no path resolution)"="LuaVIEW Retrieve Scripts_srv.vi", "error in (no error)"=w838) -> ("server app ref"=w816:refnum<vi>, "resolved server path"=w815:path, "error out"=w819:errorcluster)  [unwired: 6 in, 5 out]
        n490 = stacked-sequence {
          tunnel: [w882] -> w817
          tunnel: [w881] -> w818
          tunnel: w819 -> [w880]
          tunnel: w816 -> [w879]
          tunnel: w815 -> [w878]
          tunnel: w814 -> [w877]
          frame #0 {
            # "avoid LV8 complaints"
            n491 = Path to Array of Strings(0:w878) -> (2:w883:string[])  [unwired: 1 out]
            n492 = Array Size(array=w883) -> (size(s)=w884:i32)
            n493 = case shown="1" w884 {
              tunnel: w878 -> [w891 w897]
              tunnel: w879 -> [w889 w896]
              tunnel: [w887 w892] -> w882
              tunnel: [w885 w895] -> w881
              tunnel: w877 -> [w886 w894]
              tunnel: w880 -> [w888 w893]
              frame 1 {
                n494 = Path To String(path=w891) -> (string=w890:string)
                n495 = Open VI Reference(type specifier VI Refnum (for type only)=w886, application reference (local)=w889, vi path=w890, error in (no error)=w888) -> (vi reference=w887:T3, error out=w885:errorcluster)  [unwired: 2 in]
              }
              frame Default {
                n496 = Open VI Reference(type specifier VI Refnum (for type only)=w894, application reference (local)=w896, vi path=w897, error in (no error)=w893) -> (vi reference=w892:T3, error out=w895:errorcluster)  [unwired: 2 in]
              }
            }
          }
        }
        "retrieve scripts" <- w817
        n497 = call "Library Open VI Ref Error Clarifier.vi"("VI path"=w815, "called VI error (no error)"=w818) -> ("error out"=w840:errorcluster)  [unwired: 13 in]
        n498 = call "obj_ClientSrv Connection State.vi"("machine{connect}/VI{get state} name (local/no path resolution)"="LuaVIEW Info_srv.vi", "error in (no error)"=w840) -> ("server app ref"=w822:refnum<vi>, "resolved server path"=w821:path, "error out"=w820:errorcluster)  [unwired: 6 in, 5 out]
        n499 = local read "info"() -> (w824:T2)
        n500 = stacked-sequence {
          tunnel: [w903] -> w823
          tunnel: [w902] -> w825
          tunnel: w820 -> [w901]
          tunnel: w822 -> [w900]
          tunnel: w821 -> [w899]
          tunnel: w824 -> [w898]
          frame #0 {
            # "avoid LV8 complaints"
            n501 = Path to Array of Strings(0:w899) -> (2:w904:string[])  [unwired: 1 out]
            n502 = Array Size(array=w904) -> (size(s)=w905:i32)
            n503 = case shown="1" w905 {
              tunnel: w899 -> [w912 w918]
              tunnel: w900 -> [w910 w917]
              tunnel: [w908 w913] -> w903
              tunnel: [w906 w916] -> w902
              tunnel: w898 -> [w907 w915]
              tunnel: w901 -> [w909 w914]
              frame 1 {
                n504 = Path To String(path=w912) -> (string=w911:string)
                n505 = Open VI Reference(type specifier VI Refnum (for type only)=w907, application reference (local)=w910, vi path=w911, error in (no error)=w909) -> (vi reference=w908:T2, error out=w906:errorcluster)  [unwired: 2 in]
              }
              frame Default {
                n506 = Open VI Reference(type specifier VI Refnum (for type only)=w915, application reference (local)=w917, vi path=w918, error in (no error)=w914) -> (vi reference=w913:T2, error out=w916:errorcluster)  [unwired: 2 in]
              }
            }
          }
        }
        "info" <- w823
        n507 = call "Library Open VI Ref Error Clarifier.vi"("VI path"=w821, "called VI error (no error)"=w825) -> ("error out"=w841:errorcluster)  [unwired: 13 in]
        n508 = call "obj_ClientSrv Connection State.vi"("machine{connect}/VI{get state} name (local/no path resolution)"="obj_LuaVIEW Task List_srv.vi", "error in (no error)"=w841) -> ("server app ref"=w828:refnum<vi>, "resolved server path"=w827:path, "error out"=w826:errorcluster)  [unwired: 6 in, 5 out]
        n509 = stacked-sequence {
          tunnel: [w924] -> w829
          tunnel: [w923] -> w831
          tunnel: w826 -> [w922]
          tunnel: w828 -> [w921]
          tunnel: w827 -> [w920]
          tunnel: w830 -> [w919]
          frame #0 {
            # "avoid LV8 complaints"
            n510 = Path to Array of Strings(0:w920) -> (2:w925:string[])  [unwired: 1 out]
            n511 = Array Size(array=w925) -> (size(s)=w926:i32)
            n512 = case shown="1" w926 {
              tunnel: w920 -> [w933 w939]
              tunnel: w921 -> [w931 w938]
              tunnel: [w929 w934] -> w924
              tunnel: [w927 w937] -> w923
              tunnel: w919 -> [w928 w936]
              tunnel: w922 -> [w930 w935]
              frame 1 {
                n513 = Path To String(path=w933) -> (string=w932:string)
                n514 = Open VI Reference(type specifier VI Refnum (for type only)=w928, application reference (local)=w931, vi path=w932, error in (no error)=w930) -> (vi reference=w929:T7, error out=w927:errorcluster)  [unwired: 2 in]
              }
              frame Default {
                n515 = Open VI Reference(type specifier VI Refnum (for type only)=w936, application reference (local)=w938, vi path=w939, error in (no error)=w935) -> (vi reference=w934:T7, error out=w937:errorcluster)  [unwired: 2 in]
              }
            }
          }
        }
        "task list" <- w829
        n516 = call "Library Open VI Ref Error Clarifier.vi"("VI path"=w827, "called VI error (no error)"=w831) -> ("error out"=w848:errorcluster)  [unwired: 13 in]
        n517 = call "obj_ClientSrv Connection State.vi"("machine{connect}/VI{get state} name (local/no path resolution)"="LuaVIEW Run or Swap Task_srv.vi", "error in (no error)"=w848) -> ("server app ref"=w834:refnum<vi>, "resolved server path"=w832:path, "error out"=w833:errorcluster)  [unwired: 6 in, 5 out]
        n518 = stacked-sequence {
          tunnel: [w945] -> w836
          tunnel: [w944] -> w837
          tunnel: w833 -> [w943]
          tunnel: w834 -> [w942]
          tunnel: w832 -> [w941]
          tunnel: w835 -> [w940]
          frame #0 {
            # "avoid LV8 complaints"
            n519 = Path to Array of Strings(0:w941) -> (2:w946:string[])  [unwired: 1 out]
            n520 = Array Size(array=w946) -> (size(s)=w947:i32)
            n521 = case shown="1" w947 {
              tunnel: w941 -> [w954 w960]
              tunnel: w942 -> [w952 w959]
              tunnel: [w950 w955] -> w945
              tunnel: [w948 w958] -> w944
              tunnel: w940 -> [w949 w957]
              tunnel: w943 -> [w951 w956]
              frame 1 {
                n522 = Path To String(path=w954) -> (string=w953:string)
                n523 = Open VI Reference(type specifier VI Refnum (for type only)=w949, application reference (local)=w952, vi path=w953, error in (no error)=w951) -> (vi reference=w950:T8, error out=w948:errorcluster)  [unwired: 2 in]
              }
              frame Default {
                n524 = Open VI Reference(type specifier VI Refnum (for type only)=w957, application reference (local)=w959, vi path=w960, error in (no error)=w956) -> (vi reference=w955:T8, error out=w958:errorcluster)  [unwired: 2 in]
              }
            }
          }
        }
        "run or swap task" <- w836
        n525 = call "Library Open VI Ref Error Clarifier.vi"("VI path"=w832, "called VI error (no error)"=w837) -> ("error out"=w844:errorcluster)  [unwired: 13 in]
        n526 = call "Library Log Error to Window.vi"("error in (no error)"=w844) -> ("dup error"=w843:errorcluster)  [unwired: 13 in, 1 out]
        n527 = Select(t=w854, s=w843, f=w853) -> (s? t:f=w855:T9[])
      }
      frame "init remote dlg" {
        # "By dynamically linking to the remote file dialog and\nallowing for failure, dependency of LuaVIEW on the\nfull client-server infrastructure is avoided."
        n528 = call "obj_ClientSrv Connection State.vi"() -> ("local?"=w963:bool, "error out"=w964:errorcluster)  [unwired: 8 in, 6 out]
        n529 = case "local?" shown="False" w963 {
          tunnel: w964 -> [w972 _]
          tunnel: [w969 w977] -> w961
          frame False {
            n530 = local read "remote file dialog"() -> (w973:refnum<vi>)
            n531 = Open VI Reference(type specifier VI Refnum (for type only)=w973, vi path="ClientSrv Remote File Dialog.vi", error in (no error)=w972) -> (vi reference=→"remote file dialog":refnum<vi>, error out=w970:errorcluster)  [unwired: 3 in]
            n532 = case shown="No Error" w970 {
              tunnel: [w975 w976] -> w969
              frame No Error {
                w975 = u8 0 items=["enabled", "disabled", "grayed"] ("disabled state")
              }
              frame Error {
                w976 = u8 2 items=["enabled", "disabled", "grayed"] ("disabled state")
              }
            }
          }
          frame True {
            w977 = u8 2 items=["enabled", "disabled", "grayed"] ("disabled state")
          }
        }
        n533 = property on="run remote" class="Bool"("Disabled"=w961) -> ()  [unwired: 2 in, 2 out]
      }
      frame "init persist" {
        w980 = T9[] [enum."quick ablement", enum."resize"] items=["empty queue", "poll list", "reselect", "select", "resize", "pause task", "resume task", "stop task", "confirm error", "swap quick", "swap local", "swap remote", "kill task", "retrieve scripts", "select script", "quick ablement", "initialize", "init refs", "init remote dlg", "init persist", "init list", "init scripts", "cleanup", "stop"] ("Array Constant")
        n534 = call "Libary Persist Position and Controls.vi"("action"=enum16{"save", "load"}."load") -> ()  [unwired: 13 in, 2 out]
        n535 = Build Array (concatenate)(w980, w982) -> (w981:T9[])
      }
      frame "init list" {
        n536 = Build Array (concatenate)(t_LuaVIEW_Task_Manager_States."poll list" ("states"), w990) -> (w989:T9[])
      }
      frame "init scripts" {
        n537 = Reshape Array(w1000, 0 ("dimension size")) -> (w996:T21[])
        n538 = Reshape Array(w999, 0 ("dimension size")) -> (w994:cluster{"line numbers":i32[]}[])
        n539 = property on="script select" class="Ring (strict)"("Strings []"=string[] [], "Value"=0) -> ()  [unwired: 2 in, 2 out]
        n540 = Build Array (concatenate)(t_LuaVIEW_Task_Manager_States."select script" ("states"), w1003) -> (w1002:T9[])
      }
      frame "cleanup" {
        w1018 = T9[] [enum."stop"] items=["empty queue", "poll list", "reselect", "select", "resize", "pause task", "resume task", "stop task", "confirm error", "swap quick", "swap local", "swap remote", "kill task", "retrieve scripts", "select script", "quick ablement", "initialize", "init refs", "init remote dlg", "init persist", "init list", "init scripts", "cleanup", "stop"] ("Array Constant")
        n541 = call "obj_Library Session.vi"("method"=t_Library_Session_Methods."delist") -> ()  [unwired: 11 in, 4 out]
        n542 = call "Libary Persist Position and Controls.vi"("action"=enum16{"save", "load"}."save") -> ()  [unwired: 13 in, 2 out]
        n543 = property on="task list" class="MCListbox (strict)"("Item Names"=string[][] [], "Active Cell:Active Cell"=cluster{i32, i32} {-2, -2} ("Active Cell"), "Active Cell:Cell Background Color"=u32 15790320, "Active Cell:Active Cell"=cluster{i32, i32} {-1, -2} ("Active Cell"), "Active Cell:Cell Background Color"=u32 11776947, "Top Left Visible Cell"=cluster{"Row":u32, "Column":u32} {"Row"=0, "Column"=0}) -> ()  [unwired: 2 in, 2 out]
      }
      frame "stop" {
        n544 = Enqueue Element(queue=w1024, element=t_LuaVIEW_Task_Manager_Async_Actions."stop" ("states")) -> ()  [unwired: 2 in, 3 out]
        n545 = Reshape Array(w1026, 0 ("dimension size")) -> (w1020:T19[])
      }
    }
  }
